vi "main_003_beta.vi"() -> ()   [LabVIEW 2017]
uses:
  ISEGNHQxxu/iseg NHQ VISA Control.ctl
  <vilib>/Analysis/1siggen.llb/Ramp Pattern by Samples.vi
  <vilib>/Utility/file.llb/Read From Spreadsheet File (DBL).vi
  <vilib>/Utility/file.llb/Write Delimited Spreadsheet (string).vi
  <vilib>/Utility/file.llb/Write Delimited Spreadsheet (DBL).vi
  <vilib>/Platform/browser.llb/Open URL in Default Browser (path).vi
  <vilib>/Analysis/NI_AALBase.lvlib
  Newport ESP301/Newport ESP301.lvlib
panel:
  in  "continous acq.":bool
  in  "snap":bool
  in  "dark":bool
  in  "savebin":bool
  in  "savepng":bool
  in  "count?":bool
  in  "dark?":bool
  in  "threshold":i32=100
  in  "t_exp":dbl=0.10000637173652649 caption="Exposure time [s]"
  in  "dark_load":bool
  in  "frames":i32=300
  in  "avg[t] acc[f]":bool
  in  "Value in":dbl=2.0 caption="binning"
  in  "stop":bool
  out "Slide":dbl(slide)=0.9966666666666667 scale=0.0..1.0
  in  "open base path":bool
  in  "Path":path=path "Z:/Ediff/data/2018/08/180807"
  in  "Tab Control":T1(tab)=enum."delayscan"
  out "Waveform Chart":dbl(graph)=8402498.700000005
  in  "array size":i32=50
  out "noise-o-meter":dbl=7.252741087138157 format="%.1g"
  out "Actual Voltage":dbl[unit]=-90.03 format="%.2f"
  in  "volt_set":bool
  in  "Nominal Voltage":sgl=90.0 min=0 max=1000 step=1 format="%.2f"
  out "delayscan_time/step":dbl format="%.2f"
  out "delayscan_steps":i32
  in  "esp_rel_delta_fs":dbl=0.015 caption="delta [fs]" min=0.0
  in  "delayscan_go":bool
  in  "waypoints":string[][](table)=[["-500", "50"], ["500", ""], ["", ""]]
  in  "delayscan_header":string="DelayScan01" caption="header"
  in  "iterations":i32=1
  out "XY Graph":cluster{"Array":dbl[], dbl[]}(graph)={"Array"=[-500.0, -450.0, -400.0, -350.0, -300.0, -250.0, -200.0, -150.0, -100.0, -50.0, 0.0, 50.0, 100.0, 150.0, 200.0, 250.0, 300.0, 350.0, 400.0, 450.0, 500.0], [74.7680418855, 74.77553669695, 0.0, 0.0, 0.0, 0.0, 0.0, 0.0, 0.0, 0.0, 0.0, 0.0, 0.0, 0.0, 0.0, 0.0, 0.0, 0.0, 0.0, 0.0, 0.0]}
  in  "delayscan_stop":bool
  in  "esp_abs_dest":dbl=74.87296924580001 caption="[mm]"
  out "t0 @":dbl=74.84299 format="%.6g"
  in  "esp_set_t0":bool
  in  "esp_abs_time":dbl=200.0 caption="[fs]"
  in  "esp_rel_delta":dbl=0.015 caption="delta [mm]" min=0.0
  in  "esp_abs_go":bool
  in  "esp_rel-":bool
  in  "esp_rel+":bool
  out "delay_pos":dbl=74.77555 caption="[mm]" format="%.6g"
  out "esp_pos_fs":dbl=-449.91125160329966 caption="[fs]" format="%.6g"
  in  "delayscan_pause":bool caption="pause"
  out "duration":dbl format="%<%H:%M:%S>t"
  out "Slide 2":dbl(slide)=0.999 scale=0.0..1.0
  in  "meas_stop_volt":bool
  in  "meas_start_volt":bool
  in  "head":string="PowerVoltScan1"
  in  "volt_start":dbl format="%0.2f"
  in  "volt_end":dbl=1.0 format="%0.2f"
  in  "volt_samples":i32=128
  in  "move2com":bool
  in  "meas_start_XY":bool
  in  "showcom":bool
  in  "VISA ISEG":refnum<visa-resource-name>="COM3"
  in  "Channel (A)":enum16{"A", "B"}(ring)=enum."B"
  out "error out":errorcluster
  in  "volt_timeout":u32=6000
  in  "volt_threshold":sgl=2.0 max=4000 format="%.2f"
  in  "esp_axis":i32=1 caption="ESP Axis" min=1 max=3
  in  "esp_visa":refnum<visa-resource-name>="COM2" caption="ESP VISA"
  out "esp301":errorcluster
  in  "Serial Link (RS232)":enum16{"RS232", "USB"}(ring)
  out "captured":dbl[][](graph)
  out "live":dbl[][](graph)
  in  "close":bool
  # "camera"
  # "voltage supply"
  # "Move absolute"
  # "Move relative"
  # "Axis1"
  # "Axis2"
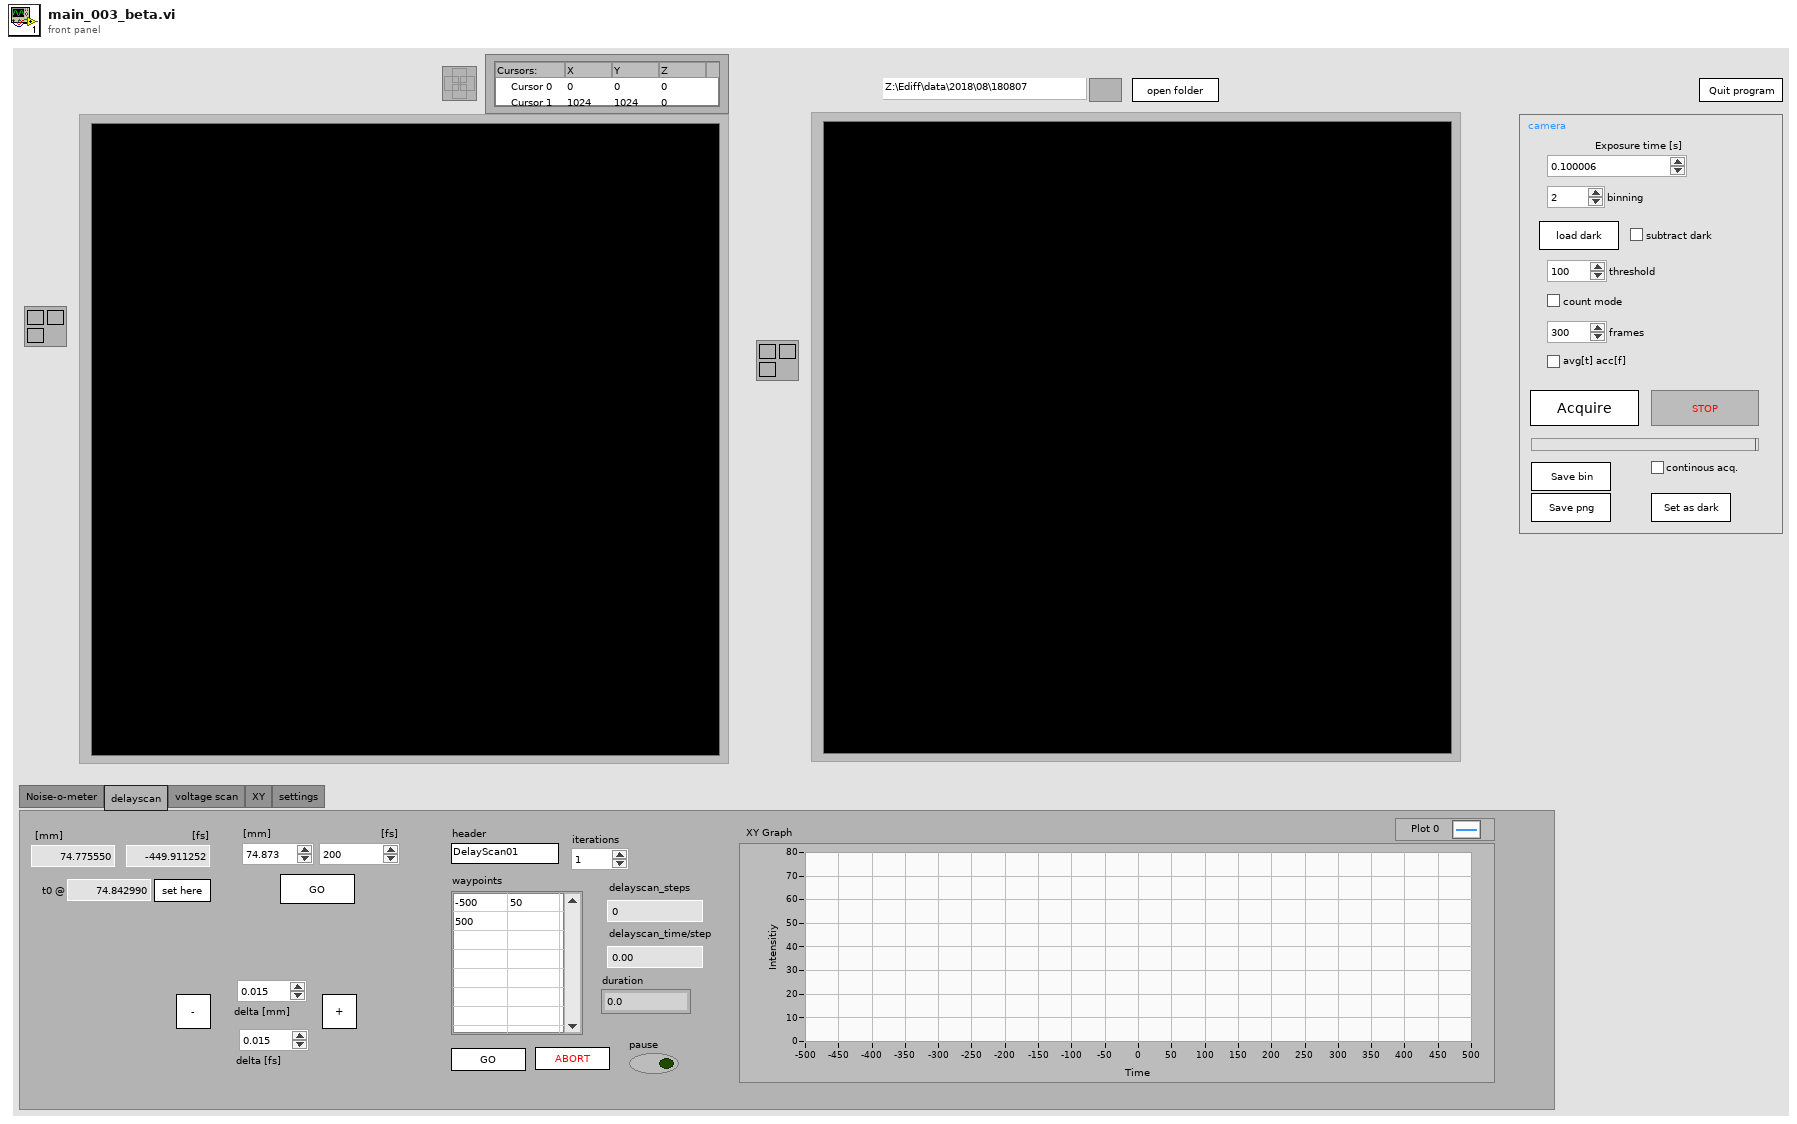
[diagram p1: front panel]
types:
  T1 = enum32{"Noise-o-meter", "delayscan", "voltage scan", "XY", "settings"}
  T2 = typedef "Image Type" = u32
  T3 = typedef "IMAQ Image.ctl" = refnum<image>
  T4 = cluster{"height":u32, "width":u32, "datatype":u32}
  T5 = cluster{"Axis1 moving":bool, "Axis2 moving":bool, "Axis3 moving":bool, "Axis4 moving":bool, "Motor Power of at least one axis":bool, "Reserved":bool, "Reserved":bool, "Reserved":bool, "Axis5 moving 2":bool, "Axis6 moving 2":bool, "Reserved":bool, "Reserved":bool, "Motor Power of at least one axis":bool, "Reserved":bool, "Reserved":bool, "Reserved":bool}
  T6 = typedef "iseg NHQ VISA Control.ctl" = cluster{"VISA Resource Name":refnum<visa-resource-name>, "FP Notation":bool, "Maximum Voltage":u32, "Maximum Current":u32}
  T7 = typedef "LVCursorListTypeDef.ctl" = cluster{"Name":string, "Color":u32, "Style":u8, "Point Style":u8, "Name Visible":bool, "Allow Drag":bool, "Cursor Mode":u32, "Plot":i32, "Index":i32, "Position":cluster{"X":dbl, "Y":dbl}, "X Scale":u32, "Y Scale":u32, "Watch Plots":i32[], "Watch All Plots":bool, "Plot Area":i32, "Label Offset":cluster{"X":dbl, "Y":dbl}}[]
  T8 = cluster{"Name":string, "Color":u32, "Style":u8, "Point Style":u8, "Name Visible":bool, "Allow Drag":bool, "Cursor Mode":u32, "Plot":i32, "Index":i32, "Position":cluster{"X":dbl, "Y":dbl}, "X Scale":u32, "Y Scale":u32, "Watch Plots":i32[], "Watch All Plots":bool, "Plot Area":i32, "Label Offset":cluster{"X":dbl, "Y":dbl}}
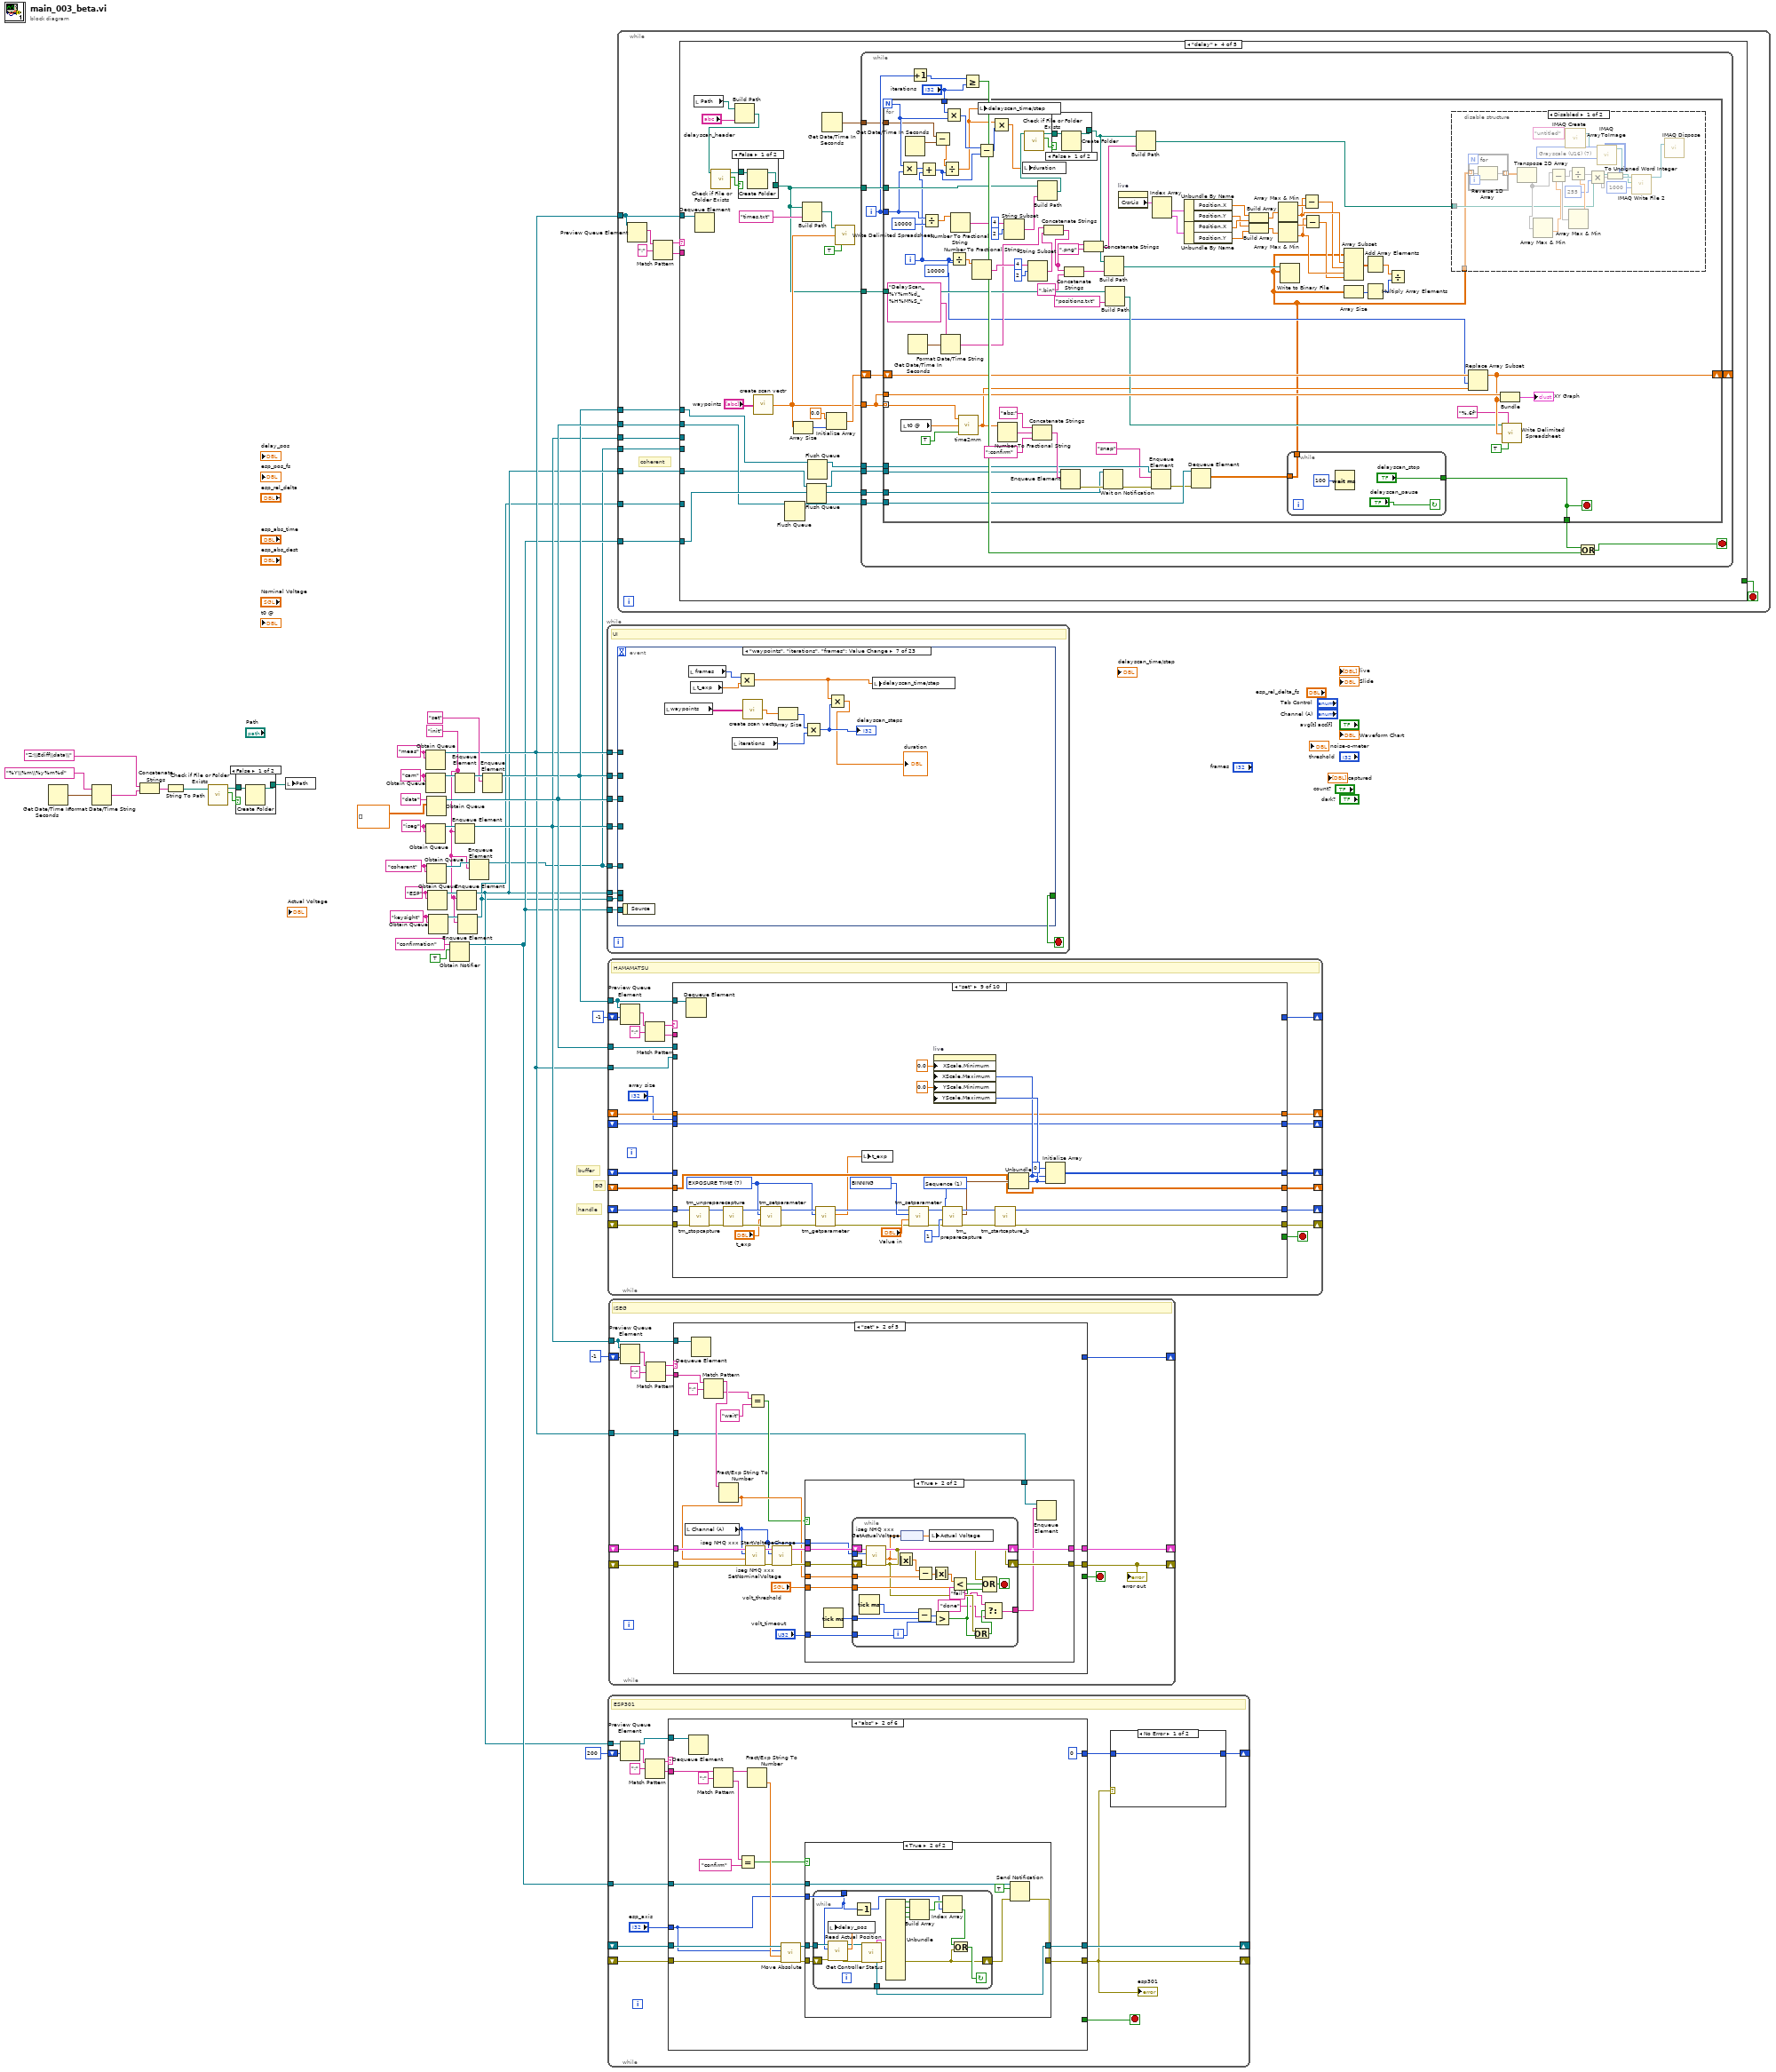
[diagram p0: block diagram]
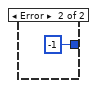
[diagram p3: hidden frame]
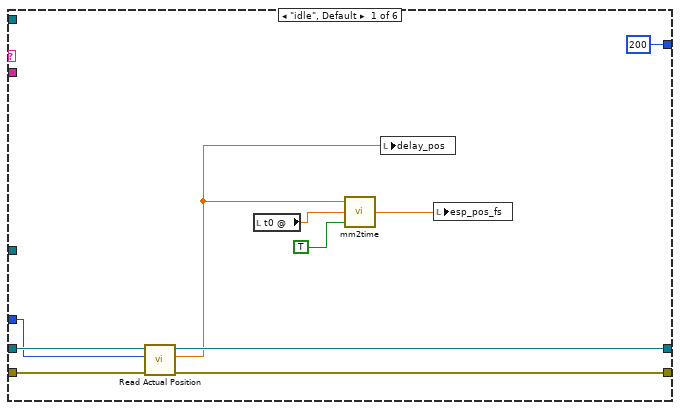
[diagram p4: hidden frame]
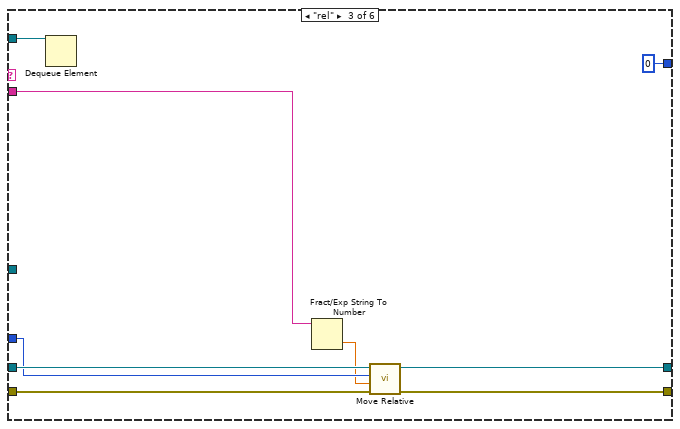
[diagram p6: hidden frame]
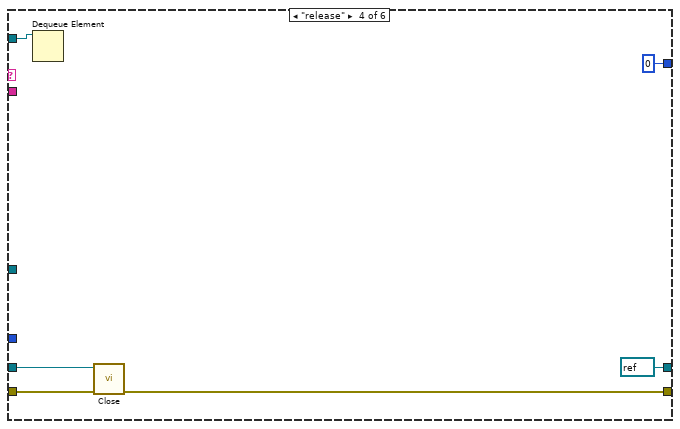
[diagram p7: hidden frame]
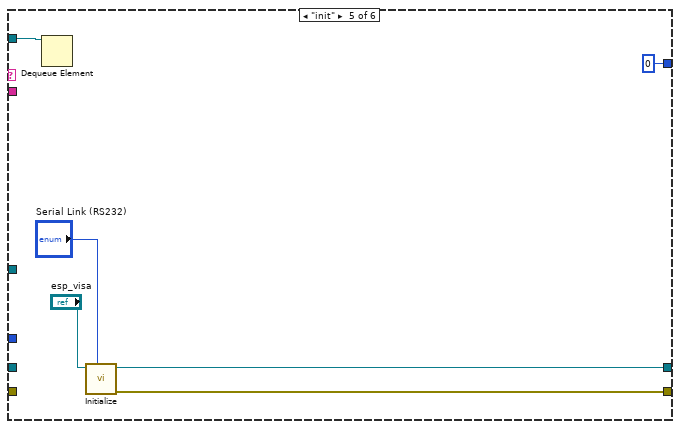
[diagram p8: hidden frame]
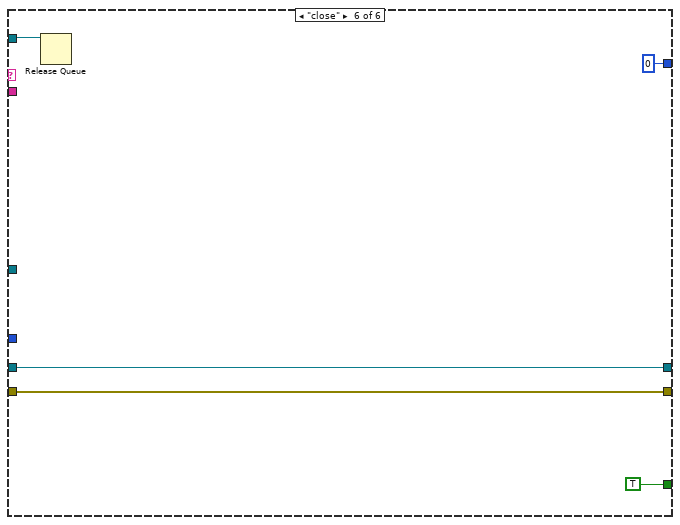
[diagram p9: hidden frame]
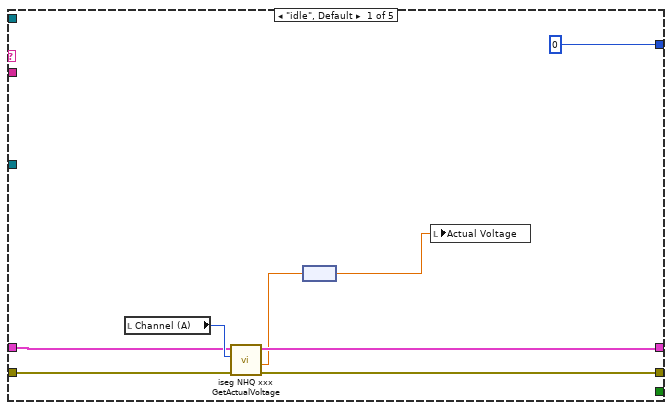
[diagram p10: hidden frame]
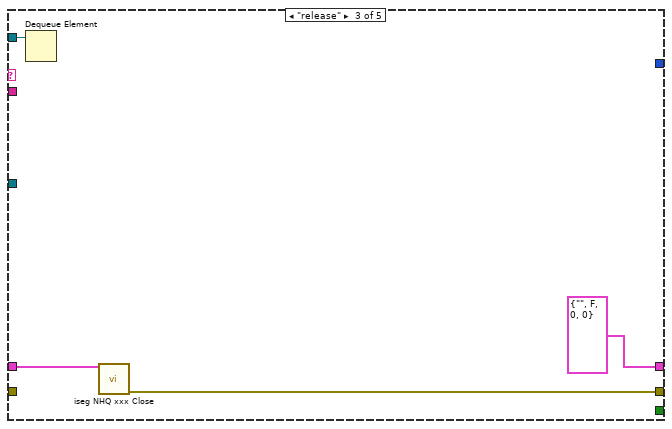
[diagram p12: hidden frame]
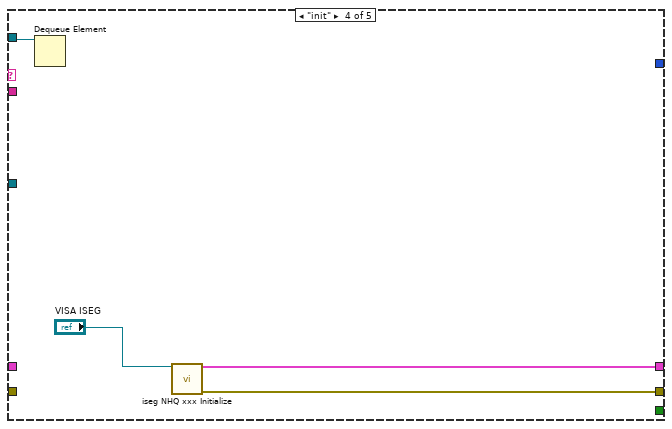
[diagram p13: hidden frame]
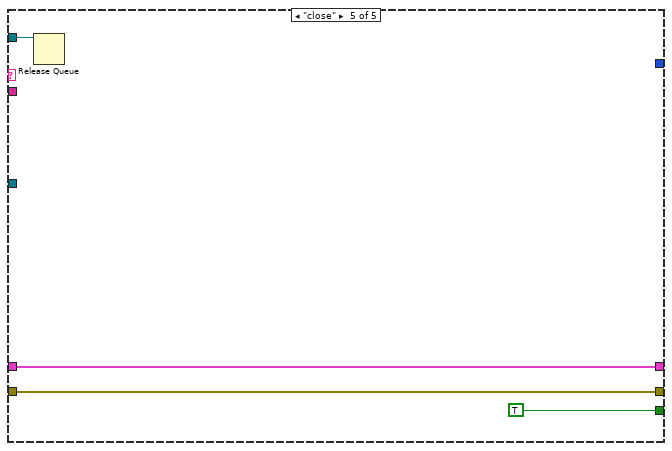
[diagram p14: hidden frame]
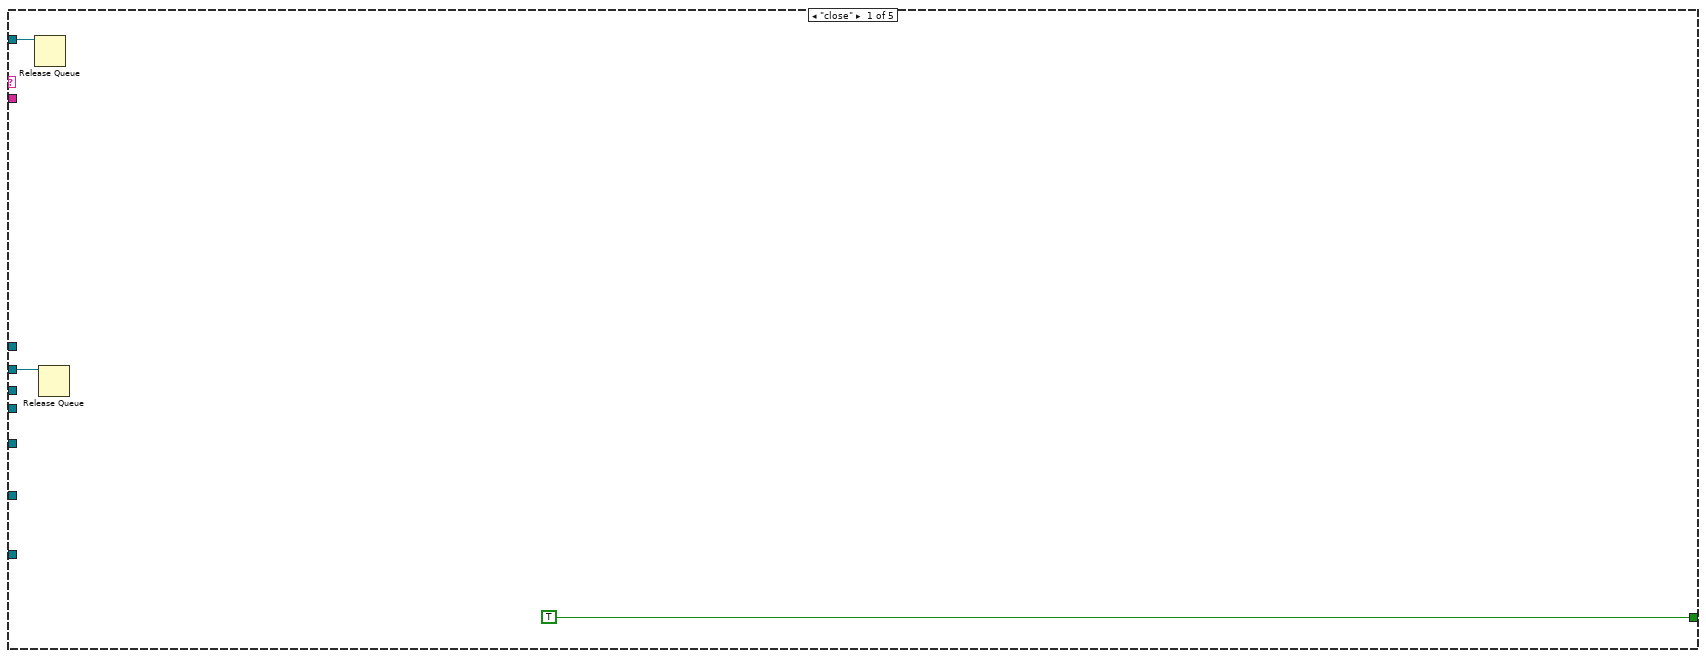
[diagram p15: hidden frame]
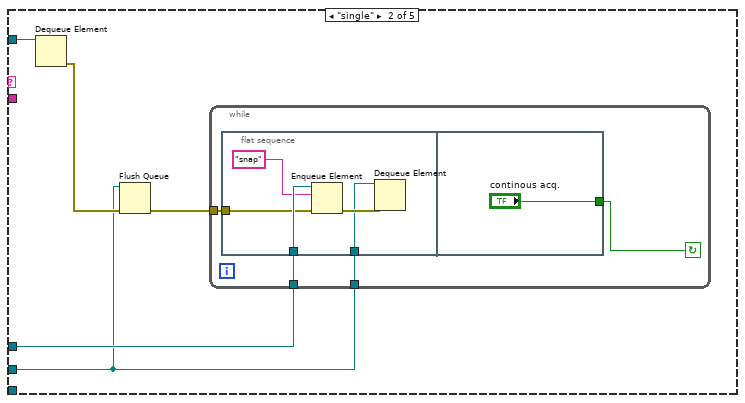
[diagram p16: hidden frame]
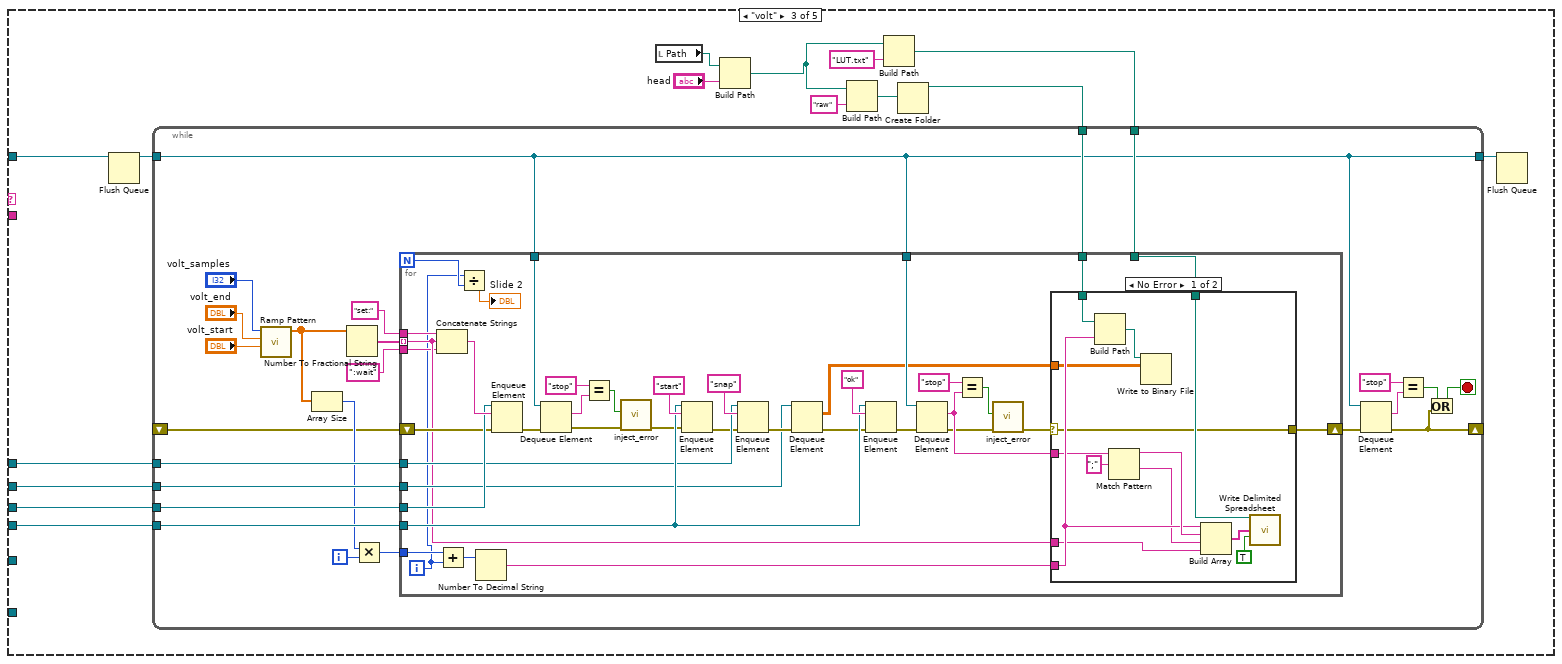
[diagram p17: hidden frame]
diagram:
  w3 = "keysight" ("name (unnamed)")
  w19 = "ESP" ("name (unnamed)")
  w24 = "coherent" ("name (unnamed)")
  w28 = "iseg" ("name (unnamed)")
  w2 = "init" ("element")
  w35 = "meas" ("name (unnamed)")
  w36 = "cam" ("name (unnamed)")
  # "BG"
  # "handle"
  # "buffer"
  n1 = Get Date/Time In Seconds() -> (seconds since 1Jan1904=w16:timestamp)
  n2 = Format Date/Time String(time format string (%c)="%Y\\%m\\%y%m%d", seconds (now)=w16) -> (date/time string=w14:string)  [unwired: 1 in]
  n3 = Concatenate Strings("Z:\\Ediff\\data\\" ("string"), w14) -> (w12:string)
  n4 = String To Path(string=w12) -> (path=w9:path)
  n5 = call <vilib>:"Check if File or Folder Exists.vi"("path"=w9) -> ("file or folder exists?"=w11:bool, "dup path"=w10:path)  [unwired: 8 in, 1 out]
  n6 = case shown="False" w11 {
    tunnel: [w40 w41] -> w8
    tunnel: w10 -> [w39 w41]
    frame False {
      n7 = Create Folder(path (use dialog)=w39) -> (created path=w40:path)  [unwired: 2 in, 2 out]
    }
    frame True {
    }
  }
  n8 = local write "Path"(w8) -> ()
  n9 = Obtain Queue(name (unnamed)=w35, element data type=w35) -> (queue out=w23:refnum<queue>)  [unwired: 3 in, 2 out]
  n10 = Obtain Queue(name (unnamed)=w36, element data type=w36) -> (queue out=w38:refnum<queue>)  [unwired: 3 in, 2 out]
  n11 = Obtain Queue(name (unnamed)=w28, element data type=w28) -> (queue out=w27:refnum<queue>)  [unwired: 3 in, 2 out]
  n12 = Obtain Queue(name (unnamed)="data", element data type=dbl[][] []) -> (queue out=w31:refnum<queue>)  [unwired: 3 in, 2 out]
  n13 = Obtain Queue(name (unnamed)=w24, element data type=w24) -> (queue out=w7:refnum<queue>)  [unwired: 3 in, 2 out]
  n14 = Obtain Queue(name (unnamed)=w19, element data type=w19) -> (queue out=w18:refnum<queue>)  [unwired: 3 in, 2 out]
  n15 = Obtain Queue(name (unnamed)=w3, element data type=w3) -> (queue out=w4:refnum<queue>)  [unwired: 3 in, 2 out]
  n16 = Obtain Notifier(name (unnamed)="confirmation", notification data type=TRUE) -> (notifier out=w20:refnum<notifier>)  [unwired: 2 in, 2 out]
  n17 = Enqueue Element(queue=w38, element=w2) -> (queue out=w34:refnum<queue>)  [unwired: 2 in, 2 out]
  n18 = Enqueue Element(queue=w27, element=w2) -> (queue out=w25:refnum<queue>)  [unwired: 2 in, 2 out]
  n19 = Enqueue Element(queue=w18, element=w2) -> (queue out=w17:refnum<queue>)  [unwired: 2 in, 2 out]
  n20 = Enqueue Element(queue=w4, element=w2) -> (queue out=w1:refnum<queue>)  [unwired: 2 in, 2 out]
  n21 = Enqueue Element(queue=w7, element=w2) -> (queue out=w6:refnum<queue>)  [unwired: 2 in, 2 out]
  n22 = Enqueue Element(queue=w34, element="set") -> (queue out=w30:refnum<queue>)  [unwired: 2 in, 2 out]
  n23 = while {
    tunnel: w30 -> [w50]
    tunnel: w23 -> [w49]
    tunnel: w31 -> [w48]
    tunnel: w25 -> [w46]
    tunnel: w6 -> [w45]
    tunnel: w20 -> [w44]
    tunnel: w17 -> [w43]
    tunnel: w1 -> [w42]
    stop <- w47 stop-if-true
    # "UI"
    n24 = event shown="[6] \"waypoints\", \"iterations\", \"frames\": Value Change" {
      selector: _ -> [_ _ _ _ _ _ _ _ _ _ _ _ _ _ _ _ _ _ _ _ _ _ _]
      dyn-events: _ -> [_ _ _ _ _ _ _ _ _ _ _ _ _ _ _ _ _ _ _ _ _ _ _]
      timeout: _ -> [_ _ _ _ _ _ _ _ _ _ _ _ _ _ _ _ _ _ _ _ _ _ _]
      tunnel: w50 -> [_ w65 _ _ _ _ _ _ _ _ _ w108 w110 _ _ _ _ _ _ w161 _ _ _]
      tunnel: w49 -> [_ w66 _ _ _ _ _ _ _ w102 _ _ _ w111 w114 w115 _ _ w155 _ w168 w170 _]
      tunnel: w48 -> [_ _ _ _ _ _ _ _ _ _ _ _ _ _ _ _ _ _ _ _ _ _ _]
      tunnel: [_ TRUE _ _ _ _ _ _ _ _ _ _ _ _ _ _ _ _ _ _ _ _ _] -> w47
      tunnel: w46 -> [_ w62 _ _ _ _ _ _ _ _ _ _ _ _ _ _ _ _ _ _ _ _ w175]
      tunnel: w45 -> [_ w59 _ _ _ _ _ _ _ _ _ _ _ _ _ _ _ _ _ _ _ _ _]
      tunnel: w44 -> [_ w56 _ _ _ _ _ _ _ _ _ _ _ _ _ _ _ _ _ _ _ _ _]
      tunnel: w43 -> [_ w58 w72 w77 _ _ _ _ _ _ _ _ _ _ _ _ _ _ _ _ _ _ _]
      tunnel: w42 -> [_ w51 _ _ _ _ _ _ _ _ _ _ _ _ _ _ _ _ _ _ _ _ _]
      event Timeout {
        n25 = event-data() -> ()  [unwired: 1 in, 1 out]
      }
      event "close": Value Change {
        w54 = "close" ("element")
        w55 = "release" ("element")
        n26 = event-data() -> ()  [unwired: 1 in, 1 out]
        n27 = Enqueue Element(queue=w59, element=w55) -> (queue out=w60:refnum<queue>)  [unwired: 2 in, 2 out]
        n28 = Enqueue Element(queue=w58, element=w55) -> (queue out=w57:refnum<queue>)  [unwired: 2 in, 2 out]
        n29 = Enqueue Element(queue=w62, element=w55) -> (queue out=w61:refnum<queue>)  [unwired: 2 in, 2 out]
        n30 = Enqueue Element(queue=w65, element=w55) -> (queue out=w64:refnum<queue>)  [unwired: 2 in, 2 out]
        n31 = Enqueue Element(queue=w66, element=w54) -> ()  [unwired: 2 in, 3 out]
        n32 = Enqueue Element(queue=w64, element=w54) -> ()  [unwired: 2 in, 3 out]
        n33 = Enqueue Element(queue=w61, element=w54) -> ()  [unwired: 2 in, 3 out]
        n34 = Enqueue Element(queue=w60, element=w54) -> ()  [unwired: 2 in, 3 out]
        n35 = Enqueue Element(queue=w57, element=w54) -> ()  [unwired: 2 in, 3 out]
        n36 = Release Notifier(notifier=w56) -> ()  [unwired: 2 in, 3 out]
        n37 = Flush Queue(queue=w51) -> (queue out=w52:refnum<queue>)  [unwired: 1 in, 2 out]
        n38 = Enqueue Element(queue=w52, element=w55) -> (queue out=w53:refnum<queue>)  [unwired: 2 in, 2 out]
        n39 = Enqueue Element(queue=w53, element=w54) -> ()  [unwired: 2 in, 3 out]
      }
      event "esp_abs_go": Value Change {
        n40 = event-data() -> ()  [unwired: 1 in, 1 out]
        n41 = local read "esp_abs_dest"() -> (w68:dbl)
        n42 = Number To Fractional String(number=w68) -> (F-format string=w69:string)  [unwired: 3 in]
        n43 = Concatenate Strings("abs:" ("string"), w69, ":confirm" ("string")) -> (w71:string)
        n44 = Enqueue Element(queue=w72, element=w71) -> ()  [unwired: 2 in, 3 out]
      }
      event "esp_rel+", "esp_rel-": Value Change {
        n45 = event-data() -> ()  [unwired: 1 in, 1 out]
        n46 = local read "esp_rel_delta"() -> (w75:dbl)
        n47 = Negate(x=w75) -> (-x=w76:dbl)
        n48 = Select(t=w76, s="esp_rel-", f=w75) -> (s? t:f=w74:dbl)
        n49 = Number To Fractional String(number=w74) -> (F-format string=w79:string)  [unwired: 3 in]
        n50 = Concatenate Strings("rel:" ("string"), w79) -> (w78:string)
        n51 = Enqueue Element(queue=w77, element=w78) -> ()  [unwired: 2 in, 3 out]
      }
      event "esp_rel_delta_fs": Value Change {
        n52 = event-data() -> ()  [unwired: 1 in, 1 out]
        n53 = local read "esp_rel_delta_fs"() -> (w81:dbl)
        n54 = call "time2mm.vi"("fs[1]/ps[0]"=TRUE, "time"=w81) -> ("position (mm)"=w82:dbl)  [unwired: 1 in]
        n55 = local write "esp_rel_delta"(w82) -> ()
      }
      event "esp_rel_delta": Value Change {
        n56 = event-data() -> ()  [unwired: 1 in, 1 out]
        n57 = local read "esp_rel_delta"() -> (w85:dbl)
        n58 = call "mm2time.vi"("fs?"=TRUE, "distance (mm)"=w85) -> ("time in fs/ps seconds"=w84:dbl)  [unwired: 1 in]
        n59 = local write "esp_rel_delta_fs"(w84) -> ()
      }
      event "waypoints", "iterations", "frames": Value Change {
        n60 = event-data() -> ()  [unwired: 1 in, 1 out]
        n61 = local read "waypoints"() -> (w95:string[][])
        n62 = local read "frames"() -> (w90:i32)
        n63 = local read "t_exp"() -> (w89:dbl)
        n64 = local read "iterations"() -> (w92:i32)
        n65 = Multiply(x=w90, y=w89) -> (x*y=w88:dbl)
        n66 = call "create scan vectr.vi"("Table Control"=w95) -> ("Array"=w94:dbl[])
        n67 = Array Size(array=w94) -> (size(s)=w93:i32)
        n68 = Multiply(x=w93, y=w92) -> (x*y=w91:i32)
        "delayscan_steps" <- w91
        n69 = Multiply(x=w88, y=w91) -> (x*y=→"duration":dbl)
        n70 = local write "delayscan_time/step"(w88) -> ()
      }
      event "esp_set_t0": Value Change {
        n71 = event-data() -> ()  [unwired: 1 in, 1 out]
        n72 = local read "delay_pos"() -> (w96:dbl)
        n73 = local write "t0 @"(w96) -> ()
      }
      event "esp_abs_time": Value Change {
        n74 = event-data() -> ()  [unwired: 1 in, 1 out]
        n75 = local read "esp_abs_time"() -> (w97:dbl)
        n76 = local read "t0 @"() -> (w98:dbl)
        n77 = call "time2mm.vi"("fs[1]/ps[0]"=TRUE, "Offset (mm)"=w98, "time"=w97) -> ("position (mm)"=w99:dbl)
        n78 = local write "esp_abs_dest"(w99) -> ()
      }
      event "delayscan_go": Value Change {
        n79 = event-data() -> ()  [unwired: 1 in, 1 out]
        n80 = Enqueue Element(queue=w102, element="delay") -> ()  [unwired: 2 in, 3 out]
      }
      event "esp_abs_dest": Value Change {
        n81 = event-data() -> ()  [unwired: 1 in, 1 out]
        n82 = local read "esp_abs_dest"() -> (w106:dbl)
        n83 = local read "t0 @"() -> (w105:dbl)
        n84 = call "mm2time.vi"("fs?"=TRUE, "Offset (mm)"=w105, "distance (mm)"=w106) -> ("time in fs/ps seconds"=w103:dbl)
        n85 = local write "esp_abs_time"(w103) -> ()
      }
      event "dark": Value Change {
        n86 = event-data() -> ()  [unwired: 1 in, 1 out]
        n87 = Enqueue Element(queue=w108, element="dark") -> ()  [unwired: 2 in, 3 out]
      }
      event "t_exp": Value Change {
        n88 = event-data() -> ()  [unwired: 1 in, 1 out]
        n89 = Enqueue Element(queue=w110, element="set") -> ()  [unwired: 2 in, 3 out]
      }
      event "snap": Value Change {
        n90 = event-data() -> ()  [unwired: 1 in, 1 out]
        n91 = Enqueue Element(queue=w111, element="single") -> ()  [unwired: 2 in, 3 out]
      }
      event "meas_start_volt": Value Change {
        n92 = event-data() -> ()  [unwired: 1 in, 1 out]
        n93 = Enqueue Element(queue=w114, element="volt") -> ()  [unwired: 2 in, 3 out]
      }
      event "meas_stop_volt": Value Change {
        n94 = event-data() -> ()  [unwired: 1 in, 1 out]
        n95 = Enqueue Element(queue=w115, element="stop") -> ()  [unwired: 2 in, 3 out]
      }
      event "open base path": Value Change {
        n96 = event-data() -> ()  [unwired: 1 in, 1 out]
        n97 = local read "Path"() -> (w117:path)
        n98 = call-poly <vilib>:"Open URL in Default Browser.vi"("path"=w117) -> ()  [unwired: 5 in, 2 out]
      }
      event "savebin", "savepng": Value Change {
        n99 = event-data() -> ()  [unwired: 1 in, 1 out]
        n100 = Get Date/Time In Seconds() -> (seconds since 1Jan1904=w123:timestamp)
        n101 = local read "Path"() -> (w119:path)
        n102 = Format Date/Time String(time format string (%c)="MCPIMG_%Y%m%d_%H%M%S", seconds (now)=w123) -> (date/time string=w118:string)  [unwired: 1 in]
        n103 = local read "captured"() -> (w120:dbl[][])
        n104 = case shown="False" "savebin" {
          tunnel: w120 -> [w138 w154]
          tunnel: w119 -> [w135 w148]
          tunnel: w118 -> [w133 w149]
          frame False {
            w143 = T2 7 items=["Grayscale (U8)", "Grayscale (I16)", "Grayscale (SGL)", "Complex (CSG)", "RGB (U32)", "HSL (U32)", "RGB (U64)", "Grayscale (U16)"] ("Image Type")
            n105 = for {
              tunnel: w138 -> [w146] mode=indexing
              tunnel: [w145] -> w137 mode=indexing
              n106 = Reverse 1D Array(array=w146) -> (reversed array=w145:dbl[])
            }
            n107 = Concatenate Strings(w133, ".png" ("string")) -> (w134:string)
            n108 = Transpose 2D Array(2D array=w137) -> (transposed array=w126:dbl[][])
            n109 = Array Max & Min(array=w126) -> (min value=w125:dbl)  [unwired: 3 out]
            n110 = Build Path(base path=w135, name or relative path=w134) -> (appended path=w136:path)
            n111 = Subtract(x=w126, y=w125) -> (x-y=w124:dbl[][])
            n112 = call "IMAQ Create"("Image Name"="untitled", "Image Type"=w143) -> ("New Image"=w144:T3)  [unwired: 3 in, 1 out]
            n113 = Array Max & Min(array=w124) -> (max value=w131:dbl)  [unwired: 3 out]
            n114 = Divide(x=w124, y=w131) -> (x/y=w130:dbl[][])
            n115 = Multiply(x=w130, y=255) -> (x*y=w128:dbl[][])
            n116 = To Unsigned Word Integer(number=w128) -> (unsigned 16bit integer=w127:u16[][])
            n117 = call "IMAQ ArrayToImage"("Image Pixels (U16)"=w127, "Image"=w144) -> ("Image Out"=w142:T3)  [unwired: 8 in, 1 out]
            n118 = call-poly "IMAQ Write File 2"("Image Quality"=u32 1000, "File Path"=w136, "Image"=w142) -> ("Image Out (duplicate)"=w140:T3)  [unwired: 7 in, 1 out]
            n119 = call "IMAQ Dispose"("Image"=w140) -> ()  [unwired: 5 in, 1 out]
          }
          frame True {
            n120 = Concatenate Strings(w149, ".bin" ("string")) -> (w151:string)
            n121 = Build Path(base path=w148, name or relative path=w151) -> (appended path=w147:path)
            n122 = Write to Binary File(file (use dialog)=w147, data=w154) -> (refnum out=w153:refnum<file>, error out=w152:errorcluster)  [unwired: 4 in, 1 out]
            n123 = Close File(refnum=w153, error in=w152) -> ()  [unwired: 2 out]
          }
        }
      }
      event "meas_start_XY": Value Change {
        n124 = event-data() -> ()  [unwired: 1 in, 1 out]
        n125 = Enqueue Element(queue=w155, element="XY") -> ()  [unwired: 2 in, 3 out]
      }
      event "dark_load": Value Change {
        n126 = event-data() -> ()  [unwired: 1 in, 1 out]
        n127 = local read "Path"() -> (w160:path)
        n128 = call "File Dialog"("start path"=w160) -> ("selected path"=w158:path, "cancelled"=w157:bool)  [unwired: 11 in, 2 out]
        n129 = case shown="False" w157 {
          tunnel: w161 -> [w166 _]
          tunnel: "dark_load:" ("element") -> [w164 _]
          tunnel: w158 -> [w162 _]
          frame False {
            n130 = Path To String(path=w162) -> (string=w163:string)
            n131 = Concatenate Strings(w164, w163) -> (w165:string)
            n132 = Enqueue Element(queue=w166, element=w165) -> ()  [unwired: 2 in, 3 out]
          }
          frame True {
          }
        }
      }
      event "move2com": Value Change {
        n133 = event-data() -> ()  [unwired: 1 in, 1 out]
        n134 = Enqueue Element(queue=w168, element="mov2cursor") -> ()  [unwired: 2 in, 3 out]
      }
      event "showcom": Value Change {
        n135 = event-data() -> ()  [unwired: 1 in, 1 out]
        n136 = Enqueue Element(queue=w170, element="showcom") -> ()  [unwired: 2 in, 3 out]
      }
      event "volt_set": Value Change {
        n137 = event-data() -> ()  [unwired: 1 in, 6 out]
        n138 = local read "Nominal Voltage"() -> (w171:sgl)
        n139 = Number To Fractional String(number=w171) -> (F-format string=w172:string)  [unwired: 3 in]
        n140 = Concatenate Strings("set:" ("element"), w172) -> (w174:string)
        n141 = Enqueue Element(queue=w175, element=w174) -> ()  [unwired: 2 in, 3 out]
      }
    }
  }
  n142 = while {
    tunnel: w30 -> [w194]
    shift-right: [w192] -> _
    shift-left: _ -> [w191]
    shift-right: [w190] -> _
    shift-left: _ -> [w189]
    shift-right: [w188] -> _
    shift-left: _ -> [w187]
    shift-right: [w186] -> _
    shift-left: _ -> [w185]
    shift-right: [w183] -> _
    shift-left: -1 -> [w184]
    tunnel: w31 -> [w182]
    tunnel: w23 -> [w181]
    shift-right: [w180] -> _
    shift-left: _ -> [w179]
    shift-right: [w177] -> _
    shift-left: _ -> [w178]
    stop <- w193 stop-if-true
    # "HAMAMATSU"
    n143 = Preview Queue Element(queue=w194, timeout in ms (-1)=w184) -> (element=w198:string)  [unwired: 1 in, 3 out]
    n144 = Match Pattern(string=w198, regular expression=":") -> (before substring=w196:string, after substring=w195:string)  [unwired: 1 in, 2 out]
    n145 = case shown="\"set\"" w196 {
      tunnel: w195 -> [_ _ w298 _ _ w388 _ _ _ _]
      tunnel: w194 -> [_ w237 w299 w333 w382 w392 w404 w407 w433 w455]
      tunnel: [_ _ _ _ _ _ _ _ _ TRUE] -> w193
      tunnel: [w217 w239 w302 w338 w380 w389 w396 w412 w421 w450] -> w192
      tunnel: w191 -> [w219 w242 w304 w340 w380 w389 w400 _ w447 w450]
      tunnel: [w218 w234 w303 w337 w379 w390 u32 0 ("Handle out") w410 w422 w451] -> w190
      tunnel: w189 -> [w220 w240 w305 w341 w379 w390 w401 _ w445 w451]
      tunnel: [w216 w241 w297 w336 w381 w391 w402 w408 w434 w452] -> w188
      tunnel: w187 -> [w216 w241 w297 w336 w381 w391 w402 w408 _ w452]
      tunnel: [w215 w238 w306 w339 w378 w385 w403 w409 w425 w453] -> w186
      tunnel: w185 -> [w215 w238 w306 w339 _ _ w403 w409 w425 w453]
      tunnel: [0 _ _ _ _ _ _ _ _ _] -> w183
      tunnel: w182 -> [_ w233 w307 _ _ _ _ _ _ _]
      tunnel: w181 -> [_ _ _ w334 _ _ _ _ _ _]
      tunnel: [w201 w228 w301 w325 w377 w384 w394 w406 w427 w449] -> w180
      tunnel: w179 -> [w210 w231 w301 w328 w377 w384 w394 w406 w427 w449]
      tunnel: w178 -> [w205 w230 w300 w326 w376 w383 w393 w405 w426 w448]
      tunnel: [w204 w227 w300 w324 w376 w383 w393 w405 w426 w448] -> w177
      tunnel: "array size" -> [w203 w229 _ w327 _ _ _ _ _ _]
      frame "idle", Default {
        n146 = local read "threshold"() -> (w221:i32)
        n147 = call "tm_getnextframe_a.vi"("error in (no error)"=w219, "Buffer"=w216, "Handle in"=w220) -> ("error out"=w217:errorcluster, "Data"=w211:u16[][], "Handle out"=w218:u32)  [unwired: 6 in]
        n148 = local read "dark?"() -> (w222:bool)
        n149 = local read "count?"() -> (w212:bool)
        n150 = case shown="False" w222 {
          tunnel: [w223 w226] -> w213
          tunnel: w211 -> [w223 w225]
          tunnel: w215 -> [_ w224]
          frame False {
          }
          frame True {
            n151 = Subtract(x=w225, y=w224) -> (x-y=w226:dbl[][])
          }
        }
        n152 = call "filtr_b.vi"("count?"=w212, "threshold"=w221, "input array"=w213) -> ("output array"=w199:dbl[][])  [unwired: 8 in]
        n153 = Add Array Elements(numeric array=w199) -> (sum=w200:dbl)
        n154 = call "ringbuffer.vi"("new val"=w200, "index in"=w205, "array size"=w203, "array in"=w210) -> ("index out"=w204:i32, "array out"=w201:dbl[])  [unwired: 6 in]
        n155 = local write "live"(w199) -> ()
        n156 = local write "Waveform Chart"(w200) -> ()
        n157 = call <vilib>:"Std Deviation and Variance.vi"("X"=w201) -> ("mean"=w206:dbl, "standard deviation"=w209:dbl)  [unwired: 1 in, 1 out]
        n158 = Divide(x=w209, y=w206) -> (x/y=w208:dbl)
        n159 = Multiply(x=w208, y=100.0) -> (x*y=w202:dbl)
        n160 = local write "noise-o-meter"(w202) -> ()
      }
      frame "snap" {
        n161 = Dequeue Element(queue=w237) -> ()  [unwired: 2 in, 4 out]
        n162 = local read "avg[t] acc[f]"() -> (w236:bool)
        n163 = local read "threshold"() -> (w244:i32)
        n164 = local read "frames"() -> (w243:i32)
        n165 = local read "count?"() -> (w235:bool)
        n166 = local read "dark?"() -> (w245:bool)
        n167 = for {
          N: w243 -> [w263]
          tunnel: w245 -> [w277]
          tunnel: w241 -> [w275]
          tunnel: w240 -> [w276]
          tunnel: w244 -> [w269]
          tunnel: [w273] -> w234
          shift-right: [w272] -> w239
          shift-left: w242 -> [w274]
          tunnel: w238 -> [w268]
          shift-right: [w246] -> w232
          shift-left: w241 -> [w266]
          tunnel: w236 -> [w267]
          tunnel: w235 -> [w265]
          shift-right: [w256] -> w228
          shift-left: w231 -> [w257]
          tunnel: w229 -> [w254]
          shift-right: [w253] -> w227
          shift-left: w230 -> [w255]
          shift-right: [w249] -> _
          shift-left: _ -> [w250]
          i -> [w264]
          stop <- "stop" stop-if-true
          n168 = call "tm_getnextframe_a.vi"("error in (no error)"=w274, "Buffer"=w275, "Handle in"=w276) -> ("error out"=w272:errorcluster, "Data"=w271:u16[][], "Handle out"=w273:u32)  [unwired: 6 in]
          n169 = Divide(x=w264, y=w263) -> (x/y=w262:dbl)
          n170 = case shown="True" w277 {
            tunnel: [w288 w291] -> w270
            tunnel: w271 -> [w288 w290]
            tunnel: w268 -> [_ w289]
            frame False {
            }
            frame True {
              n171 = Subtract(x=w290, y=w289) -> (x-y=w291:dbl[][])
            }
          }
          n172 = local write "Slide"(w262) -> ()
          n173 = Tick Count (ms)() -> (millisecond timer value=w249:u32)
          n174 = call "filtr_b.vi"("count?"=w265, "threshold"=w269, "input array"=w270) -> ("output array"=w248:dbl[][])  [unwired: 8 in]
          n175 = Subtract(x=w249, y=w250) -> ()  [unwired: 1 out]
          n176 = Add Array Elements(numeric array=w248) -> (sum=w247:dbl)
          n177 = call "ringbuffer.vi"("new val"=w247, "index in"=w255, "array size"=w254, "array in"=w257) -> ("index out"=w253:i32, "array out"=w256:dbl[])  [unwired: 6 in]
          n178 = call <vilib>:"Std Deviation and Variance.vi"("X"=w256) -> ("mean"=w258:dbl, "standard deviation"=w260:dbl)  [unwired: 1 in, 1 out]
          n179 = local write "live"(w248) -> ()
          n180 = local write "Waveform Chart"(w247) -> ()
          n181 = Divide(x=w260, y=w258) -> (x/y=w252:dbl)
          n182 = case shown="True" w267 {
            tunnel: w266 -> [w280 w287]
            tunnel: w248 -> [w279 w285]
            tunnel: [w278 w281] -> w246
            tunnel: w264 -> [_ w282]
            frame False {
              n183 = Add(x=w280, y=w279) -> (x+y=w278:dbl[][])
            }
            frame True {
              n184 = Multiply(x=w287, y=w282) -> (x*y=w286:dbl[][])
              n185 = Increment(x=w282) -> (x+1=w283:i32)
              n186 = Add(x=w286, y=w285) -> (x+y=w284:dbl[][])
              n187 = Divide(x=w284, y=w283) -> (x/y=w281:dbl[][])
            }
          }
          n188 = Multiply(x=w252, y=100.0) -> (x*y=w251:dbl)
          n189 = local write "noise-o-meter"(w251) -> ()
          n190 = local write "captured"(w246) -> ()
        }
        n191 = local write "captured"(w232) -> ()
        n192 = Enqueue Element(queue=w233, element=w232) -> ()  [unwired: 2 in, 3 out]
      }
      frame "single" {
        n193 = Dequeue Element(queue=w299) -> ()  [unwired: 2 in, 4 out]
        n194 = Decimal String To Number(string=w298) -> (number=w293:i32)  [unwired: 2 in, 1 out]
        n195 = To Unsigned Quad Integer(1:w297) -> (0:w296:u64[][])
        n196 = for {
          N: w293 -> [_]
          tunnel: w297 -> [w319]
          tunnel: w305 -> [w318]
          tunnel: w304 -> [w317]
          tunnel: [w316] -> w303
          tunnel: [w315] -> w302
          shift-right: [w312] -> w295
          shift-left: w296 -> [w314]
          n197 = call "tm_getnextframe_a.vi"("error in (no error)"=w317, "Buffer"=w319, "Handle in"=w318) -> ("error out"=w315:errorcluster, "Data"=w313:u16[][], "Handle out"=w316:u32)  [unwired: 6 in]
          n198 = Add(x=w313, y=w314) -> (x+y=w312:u64[][])
        }
        n199 = local read "dark?"() -> (w308:bool)
        n200 = Divide(x=w295, y=w293) -> (x/y=w294:dbl[][])
        n201 = case shown="True" w308 {
          tunnel: [w320 w323] -> w311
          tunnel: w294 -> [w320 w322]
          tunnel: w306 -> [_ w321]
          frame False {
          }
          frame True {
            n202 = Subtract(x=w322, y=w321) -> (x-y=w323:dbl[][])
          }
        }
        n203 = local read "threshold"() -> (w309:i32)
        n204 = local read "count?"() -> (w310:bool)
        n205 = call "filtr_b.vi"("count?"=w310, "threshold"=w309, "input array"=w311) -> ("output array"=w292:dbl[][])  [unwired: 8 in]
        n206 = Enqueue Element(queue=w307, element=w292) -> ()  [unwired: 2 in, 3 out]
        n207 = local write "captured"(w292) -> ()
      }
      frame "snap_I" {
        n208 = Dequeue Element(queue=w333) -> ()  [unwired: 2 in, 4 out]
        n209 = local read "threshold"() -> (w344:i32)
        n210 = local read "frames"() -> (w343:i32)
        n211 = local read "count?"() -> (w342:bool)
        n212 = local read "dark?"() -> (w345:bool)
        n213 = for {
          N: w343 -> [w359]
          tunnel: w345 -> [w371]
          tunnel: w336 -> [w369]
          tunnel: w341 -> [w370]
          tunnel: w344 -> [w363]
          tunnel: [w367] -> w337
          shift-right: [w366] -> w338
          shift-left: w340 -> [w368]
          tunnel: w339 -> [w362]
          tunnel: w342 -> [w361]
          tunnel: [w357] -> w335 mode=indexing
          shift-right: [w349] -> w325
          shift-left: w328 -> [w350]
          tunnel: w327 -> [w348]
          shift-right: [w346] -> w324
          shift-left: w326 -> [w347]
          i -> [w360]
          n214 = call "tm_getnextframe_a.vi"("error in (no error)"=w368, "Buffer"=w369, "Handle in"=w370) -> ("error out"=w366:errorcluster, "Data"=w365:u16[][], "Handle out"=w367:u32)  [unwired: 6 in]
          n215 = call "ringbuffer.vi"("index in"=w347, "array size"=w348, "array in"=w350) -> ("index out"=w346:i32, "array out"=w349:dbl[])  [unwired: 7 in]
          n216 = Divide(x=w360, y=w359) -> (x/y=w358:dbl)
          n217 = case shown="True" w371 {
            tunnel: [w372 w375] -> w364
            tunnel: w365 -> [w372 w374]
            tunnel: w362 -> [_ w373]
            frame False {
            }
            frame True {
              n218 = Subtract(x=w374, y=w373) -> (x-y=w375:dbl[][])
            }
          }
          n219 = local write "Slide"(w358) -> ()
          n220 = call <vilib>:"Std Deviation and Variance.vi"("X"=w349) -> ("mean"=w351:dbl, "standard deviation"=w354:dbl)  [unwired: 1 in, 1 out]
          n221 = call "filtr_b.vi"("count?"=w361, "threshold"=w363, "input array"=w364) -> ("output array"=w356:dbl[][])  [unwired: 8 in]
          n222 = Divide(x=w354, y=w351) -> (x/y=w353:dbl)
          n223 = local write "live"(w356) -> ()
          n224 = Multiply(x=w353, y=100.0) -> (x*y=w355:dbl)
          n225 = local write "noise-o-meter"(w355) -> ()
          n226 = Add Array Elements(numeric array=w356) -> (sum=w357:dbl)
          n227 = local write "Waveform Chart"(w357) -> ()
        }
        n228 = call <vilib>:"Std Deviation and Variance.vi"("X"=w335) -> ("mean"=w332:dbl, "standard deviation"=w331:dbl)  [unwired: 1 in, 1 out]
        n229 = Format Into String(format string="%.6e;%.6e", w332, w331) -> (resulting string=w330:string)  [unwired: 2 in, 1 out]
        n230 = Enqueue Element(queue=w334, element=w330) -> ()  [unwired: 2 in, 3 out]
      }
      frame "dark" {
        n231 = Dequeue Element(queue=w382) -> ()  [unwired: 2 in, 4 out]
        n232 = local read "captured"() -> (w378:dbl[][])
      }
      frame "dark_load" {
        n233 = Dequeue Element(queue=w392) -> ()  [unwired: 2 in, 4 out]
        n234 = String To Path(string=w388) -> (path=w387:path)
        n235 = Read from Binary File(5:dbl[][] [] ("all rows"), 11:w387) -> (2:w385:dbl[][])  [unwired: 4 in, 3 out]
        n236 = call-poly <vilib>:"Read From Spreadsheet File.vi"("file path (dialog if empty)"=w387) -> ()  [unwired: 6 in, 5 out]
      }
      frame "release" {
        n237 = call "tm_stopcapture.vi"("error in (no error)"=w400, "Handle in"=w401) -> ("error out"=w398:errorcluster, "Handle out"=w399:u32)  [unwired: 8 in]
        n238 = Dequeue Element(queue=w404) -> ()  [unwired: 2 in, 4 out]
        n239 = call "tm_closecamera.vi"("error in (no error)"=w398, "Handle in"=w399) -> ("error out"=w397:errorcluster)  [unwired: 9 in]
        n240 = call "tm_deinitialize.vi"("error in (no error)"=w397) -> ("error out"=w396:errorcluster)  [unwired: 10 in]
      }
      frame "init" {
        n241 = Dequeue Element(queue=w407) -> ()  [unwired: 2 in, 4 out]
        n242 = call "tm_initialize.vi"() -> ("error out"=w413:errorcluster)  [unwired: 8 in, 3 out]
        n243 = call "tm_opencamera.vi"("error in (no error)"=w413, "Camera Index"=u32 0) -> ("error out"=w412:errorcluster, "Handle out"=w410:u32)  [unwired: 7 in, 1 out]
      }
      frame "set" {
        w439 = 1 items=["Snap", "Sequence"] ("Capture mode")
        w440 = u32 4215968 items=["BINNING"=4215968, "BITS PER CHANNEL"=2, "ACTIVE VIEW INDEX"=3, "CCD MODE"=4, "SENSOR MODE"=5, "READOUT MODE"=6, "EXPOSURE TIME"=7, "CONTRAST GAIN"=8, "CONTRAST OFFSET"=9, "LIGHT MODE"=10, "SENSITIVITY"=11, "WHITE BALANCE"=12, "PHOTON IMAGING MODE"=13, "HIGH DYNAMIC RANGE MODE"=14, "TRIGGER SOURCE"=15, "TRIGGER ACTIVE"=16, "TRIGGER MODE"=17, "TRIGGER POLARITY"=18, "TRIGGER GLOBAL EXPOSURE"=19, "FIRST TRIGGER BEHAVIOR"=20, "TRIGGER TIMES"=21, "OUTPUT TRIGGER POLARITY"=22, "OUTPUT TRIGGER DELAY"=23, "OUTPUT TRIGGER PERIOD"=24, "TEMPERATURE"=25, "TEMPERATURE TARGET"=26, "SENSOR COOLER FAN"=27, "MECHANICAL SHUTTER"=28, "BACK FOCUS POSITION"=29, "FRAMEBUNDLE MODE"=30, "FRAMEBUNDLE NUMBER"=31, "LINEBUNDLE HEIGHT"=32, "TRIGGER CONNECTOR"=33, "IMAGE PIXEL TYPE"=34, "OUTPUT TRIGGER KIND"=35, "READOUT DIRECTION"=36, "CHANNEL SYNC"=37] ("Parameter")
        w417 = u32 7 items=["BINNING"=4215968, "BITS PER CHANNEL"=2, "ACTIVE VIEW INDEX"=3, "CCD MODE"=4, "SENSOR MODE"=5, "READOUT MODE"=6, "EXPOSURE TIME"=7, "CONTRAST GAIN"=8, "CONTRAST OFFSET"=9, "LIGHT MODE"=10, "SENSITIVITY"=11, "WHITE BALANCE"=12, "PHOTON IMAGING MODE"=13, "HIGH DYNAMIC RANGE MODE"=14, "TRIGGER SOURCE"=15, "TRIGGER ACTIVE"=16, "TRIGGER MODE"=17, "TRIGGER POLARITY"=18, "TRIGGER GLOBAL EXPOSURE"=19, "FIRST TRIGGER BEHAVIOR"=20, "TRIGGER TIMES"=21, "OUTPUT TRIGGER POLARITY"=22, "OUTPUT TRIGGER DELAY"=23, "OUTPUT TRIGGER PERIOD"=24, "TEMPERATURE"=25, "TEMPERATURE TARGET"=26, "SENSOR COOLER FAN"=27, "MECHANICAL SHUTTER"=28, "BACK FOCUS POSITION"=29, "FRAMEBUNDLE MODE"=30, "FRAMEBUNDLE NUMBER"=31, "LINEBUNDLE HEIGHT"=32, "TRIGGER CONNECTOR"=33, "IMAGE PIXEL TYPE"=34, "OUTPUT TRIGGER KIND"=35, "READOUT DIRECTION"=36, "CHANNEL SYNC"=37] ("Parameter")
        n244 = Dequeue Element(queue=w433) -> ()  [unwired: 2 in, 4 out]
        n245 = call "tm_stopcapture.vi"("error in (no error)"=w447, "Handle in"=w445) -> ("error out"=w446:errorcluster, "Handle out"=w444:u32)  [unwired: 8 in]
        n246 = call "tm_unpreparecapture.vi"("error in (no error)"=w446, "Handle in"=w444) -> ("error out"=w443:errorcluster, "Handle out"=w442:u32)  [unwired: 8 in]
        n247 = call "tm_setparameter.vi"("error in (no error)"=w443, "Value in"="t_exp", "Parameter"=w417, "Handle in"=w442) -> ("error out"=w419:errorcluster, "Handle out"=w418:u32)  [unwired: 6 in]
        n248 = call "tm_getparameter.vi"("error in (no error)"=w419, "Parameter"=w417, "Handle in"=w418) -> ("error out"=w415:errorcluster, "Value out"=w414:dbl, "Handle out"=w416:u32)  [unwired: 6 in]
        n249 = local write "t_exp"(w414) -> ()
        n250 = call "tm_setparameter.vi"("error in (no error)"=w415, "Value in"="Value in", "Parameter"=w440, "Handle in"=w416) -> ("error out"=w423:errorcluster, "Handle out"=w424:u32)  [unwired: 6 in]
        n251 = call "tm_preparecapture.vi"("error in (no error)"=w423, "Frames"=1, "Capture mode"=w439, "Handle in"=w424) -> ("error out"=w436:errorcluster, "Buffer Info"=w435:T4, "Handle out"=w437:u32)  [unwired: 4 in, 1 out]
        n252 = call "tm_startcapture_b.vi"("error in (no error)"=w436, "Handle in"=w437) -> ("error out"=w421:errorcluster, "Handle out"=w422:u32)  [unwired: 8 in]
        n253 = Unbundle(w435) -> ("height"=w431:u32, "width"=w432:u32)  [unwired: 1 out]
        n254 = property on="live" class="IntGraph (strict)"("XScale.Minimum"=0.0 ("X Scale.Range:Minimum"), "XScale.Maximum"=w431, "YScale.Minimum"=0.0 ("Y Scale.Range:Minimum"), "YScale.Maximum"=w432) -> ()  [unwired: 2 in, 2 out]
        n255 = Initialize Array(u16 0 ("element"), w431, w432) -> (w434:u16[][])
      }
      frame "close" {
        n256 = Release Queue(queue=w455) -> ()  [unwired: 2 in, 3 out]
      }
    }
  }
  n257 = while {
    shift-right: [w458] -> _
    shift-left: _ -> [w466]
    shift-right: [w464] -> _
    shift-left: 200 -> [w465]
    shift-right: [w462] -> _
    shift-left: _ -> [w461]
    tunnel: w20 -> [w459]
    tunnel: w17 -> [w456]
    stop <- w467 stop-if-true
    # "ESP301"
    n258 = Preview Queue Element(queue=w456, timeout in ms (-1)=w465) -> (queue out=w463:refnum<queue>, element=w471:string)  [unwired: 1 in, 2 out]
    n259 = Match Pattern(string=w471, regular expression=":") -> (before substring=w469:string, after substring=w468:string)  [unwired: 1 in, 2 out]
    n260 = case shown="\"abs\"" w469 {
      tunnel: w468 -> [_ w496 w536 _ _ _]
      tunnel: [_ _ _ _ _ TRUE] -> w467
      tunnel: [w480 w491 w532 w539 w547 w552] -> w458
      tunnel: w466 -> [w483 w500 w534 w541 _ w552]
      tunnel: w463 -> [_ w487 w528 w538 w548 w550]
      tunnel: [w481 w484 w533 refnum<visa-resource-name> refnum ("VISA resource name out") w546 w551] -> w462
      tunnel: w461 -> [w482 w499 w535 w542 _ w551]
      tunnel: "esp_axis" -> [w479 w485 w531 _ _ _]
      tunnel: w459 -> [_ w489 _ _ _ _]
      tunnel: [200 0 0 0 0 0] -> w457
      frame "idle", Default {
        n261 = call "Read Actual Position.vi"("error in (no error)"=w483, "Axis (1)"=w479, "VISA resource name"=w482) -> ("error out"=w480:errorcluster, "Position (units)"=w474:dbl, "VISA resource name out"=w481:refnum<visa-resource-name>)  [unwired: 2 in]
        n262 = local read "t0 @"() -> (w477:dbl)
        n263 = call "mm2time.vi"("fs?"=TRUE, "Offset (mm)"=w477, "distance (mm)"=w474) -> ("time in fs/ps seconds"=w475:dbl)
        n264 = local write "delay_pos"(w474) -> ()
        n265 = local write "esp_pos_fs"(w475) -> ()
      }
      frame "abs" {
        n266 = Dequeue Element(queue=w487) -> ()  [unwired: 2 in, 4 out]
        n267 = Match Pattern(string=w496, regular expression=":") -> (before substring=w495:string, after substring=w494:string)  [unwired: 1 in, 2 out]
        n268 = Equal?(x=w494, y="confirm") -> (x = y?=w490:bool)
        n269 = Fract/Exp String To Number(string=w495) -> (number=w498:dbl)  [unwired: 3 in, 1 out]
        n270 = call "Move Absolute.vi"("error in (no error)"=w500, "Position (0 units)"=w498, "Axis (1)"=w485, "VISA resource name"=w499) -> ("error out"=w492:errorcluster, "VISA resource name out"=w486:refnum<visa-resource-name>)  [unwired: 2 in]
        n271 = case shown="True" w490 {
          tunnel: w492 -> [w502 w507]
          tunnel: [w502 w510] -> w491
          tunnel: w489 -> [_ w509]
          tunnel: w486 -> [w501 w505]
          tunnel: w485 -> [_ w504]
          tunnel: [w501 w503] -> w484
          frame False {
          }
          frame True {
            n272 = while {
              tunnel: w505 -> [w515]
              tunnel: w504 -> [w511]
              shift-right: [w519] -> w506
              shift-left: w507 -> [w514]
              tunnel: [w518] -> w503
              stop <- w521 continue-if-true
              n273 = call "Read Actual Position.vi"("error in (no error)"=w514, "Axis (1)"=w511, "VISA resource name"=w515) -> ("error out"=w512:errorcluster, "Position (units)"=w516:dbl, "VISA resource name out"=w513:refnum<visa-resource-name>)  [unwired: 2 in]
              n274 = local write "delay_pos"(w516) -> ()
              n275 = Decrement(x=w511) -> (x-1=w517:i32)
              n276 = call "Get Controller Status.vi"("error in (no error)"=w512, "VISA resource name"=w513) -> ("error out"=w519:errorcluster, "Controller Status"=w527:T5, "VISA resource name out"=w518:refnum<visa-resource-name>)  [unwired: 2 in, 1 out]
              n277 = Unbundle(w527) -> ("Axis1 moving"=w526:bool, "Axis2 moving"=w525:bool, "Axis3 moving"=w524:bool, "Axis4 moving"=w523:bool)  [unwired: 12 out]
              n278 = Build Array(w526, w525, w524, w523) -> (w522:bool[])
              n279 = Index Array(array=w522, index=w517) -> (element=w520:bool)
              n280 = Or(x=w520, y=w519) -> (x .or. y?=w521:bool)
            }
            n281 = Send Notification(notification=TRUE, notifier=w509, error in (no error)=w506) -> (error out=w510:errorcluster)  [unwired: 1 out]
          }
        }
      }
      frame "rel" {
        n282 = Dequeue Element(queue=w528) -> ()  [unwired: 2 in, 4 out]
        n283 = Fract/Exp String To Number(string=w536) -> (number=w530:dbl)  [unwired: 3 in, 1 out]
        n284 = call "Move Relative.vi"("error in (no error)"=w534, "Position (0 units)"=w530, "Axis (1)"=w531, "VISA resource name"=w535) -> ("error out"=w532:errorcluster, "VISA resource name out"=w533:refnum<visa-resource-name>)  [unwired: 2 in]
      }
      frame "release" {
        n285 = Dequeue Element(queue=w538) -> ()  [unwired: 2 in, 4 out]
        n286 = call "Close.vi"("error in (no error)"=w541, "VISA resource name"=w542) -> ("error out"=w539:errorcluster)  [unwired: 9 in]
      }
      frame "init" {
        n287 = Dequeue Element(queue=w548) -> ()  [unwired: 2 in, 4 out]
        n288 = call "Initialize.vi"("VISA resource name"="esp_visa", "Serial Link (RS232)"="Serial Link (RS232)") -> ("VISA resource name out"=w546:refnum<visa-resource-name>, "error out"=w547:errorcluster)  [unwired: 7 in]
      }
      frame "close" {
        n289 = Release Queue(queue=w550) -> ()  [unwired: 2 in, 3 out]
      }
    }
    "esp301" <- w458
    n290 = case shown="No Error" w458 {
      tunnel: [w472 -1] -> w464
      tunnel: w457 -> [w472 _]
      frame No Error {
      }
      frame Error {
      }
    }
  }
  n291 = while {
    tunnel: w25 -> [w562]
    shift-right: [w560] -> _
    shift-left: _ -> [w559]
    shift-right: [w557] -> _
    shift-left: -1 -> [w558]
    shift-right: [w556] -> _
    shift-left: _ -> [w555]
    tunnel: w23 -> [w554]
    stop <- w561 stop-if-true
    # "ISEG"
    n292 = Preview Queue Element(queue=w562, timeout in ms (-1)=w558) -> (element=w566:string)  [unwired: 1 in, 3 out]
    n293 = Match Pattern(string=w566, regular expression=":") -> (before substring=w564:string, after substring=w563:string)  [unwired: 1 in, 2 out]
    n294 = case shown="\"set\"" w564 {
      tunnel: w563 -> [_ w580 _ _ _]
      tunnel: w562 -> [_ w592 w634 w638 w642]
      tunnel: [_ _ _ _ TRUE] -> w561
      tunnel: [w569 w586 w632 w637 w639] -> w560
      tunnel: w559 -> [w571 w590 _ _ w639]
      tunnel: [0 _ _ _ _] -> w557
      tunnel: [w570 w587 T6 {"VISA Resource Name"="", "FP Notation"=FALSE, "Maximum Voltage"=0, "Maximum Current"=0} ("VISA Session Out") w635 w640] -> w556
      tunnel: w555 -> [w572 w591 w633 _ w640]
      tunnel: w554 -> [_ w575 _ _ _]
      frame "idle", Default {
        n295 = local read "Channel (A)"() -> (w573:enum16{"A", "B"})
        n296 = call "iseg NHQ xxx GetActualVoltage.vi"("error in (no error)"=w571, "Channel (A)"=w573, "VISA Session"=w572) -> ("error out"=w569:errorcluster, "Voltage"=w568:dbl, "VISA Session Out"=w570:T6)  [unwired: 5 in, 1 out]
        n297 = node(w568) -> (w567:dbl[unit])
        n298 = local write "Actual Voltage"(w567) -> ()
      }
      frame "set" {
        n299 = local read "Channel (A)"() -> (w583:enum16{"A", "B"})
        n300 = Dequeue Element(queue=w592) -> ()  [unwired: 2 in, 4 out]
        n301 = Match Pattern(string=w580, regular expression=":") -> (before substring=w579:string, after substring=w578:string)  [unwired: 1 in, 2 out]
        n302 = Fract/Exp String To Number(string=w579) -> (number=w582:dbl)  [unwired: 3 in, 1 out]
        n303 = call "iseg NHQ xxx SetNominalVoltage.vi"("error in (no error)"=w590, "Voltage (0 V)"=w582, "Channel (A)"=w583, "VISA Session"=w591) -> ("error out"=w593:errorcluster, "VISA Session Out"=w594:T6)  [unwired: 6 in]
        n304 = Equal?(x=w578, y="wait") -> (x = y?=w576:bool)
        n305 = call "iseg NHQ xxx StartVoltageChange.vi"("error in (no error)"=w593, "Channel (A)"=w583, "VISA Session"=w594) -> ("error out"=w588:errorcluster, "VISA Session Out"=w589:T6)  [unwired: 6 in, 1 out]
        n306 = case shown="True" w576 {
          tunnel: [w596 w606] -> w587
          tunnel: [w595 w598] -> w586
          tunnel: w589 -> [w596 w605]
          tunnel: w588 -> [w595 w604]
          tunnel: w582 -> [_ w603]
          tunnel: "volt_threshold" -> [_ w602]
          tunnel: "volt_timeout" -> [_ w601]
          tunnel: w583 -> [_ w600]
          tunnel: w575 -> [_ w599]
          frame False {
          }
          frame True {
            n307 = Tick Count (ms)() -> (millisecond timer value=w607:u32)
            n308 = while {
              shift-right: [w628] -> w606
              shift-left: w605 -> [w630]
              shift-right: [w615] -> w598
              shift-left: w604 -> [w629]
              tunnel: w600 -> [w627]
              tunnel: w602 -> [w624]
              tunnel: w607 -> [w622]
              tunnel: w601 -> [w620]
              tunnel: w603 -> [w619]
              tunnel: [w610] -> w597
              stop <- w616 stop-if-true
              n309 = Tick Count (ms)() -> (millisecond timer value=w623:u32)
              n310 = call "iseg NHQ xxx GetActualVoltage.vi"("error in (no error)"=w629, "Channel (A)"=w627, "VISA Session"=w630) -> ("error out"=w615:errorcluster, "Voltage"=w608:dbl, "VISA Session Out"=w628:T6)  [unwired: 5 in, 1 out]
              n311 = Absolute Value(x=w608) -> (abs(x)=w618:dbl)
              n312 = node(w608) -> (w609:dbl[unit])
              n313 = Subtract(x=w623, y=w622) -> (x-y=w621:u32)
              n314 = Subtract(x=w618, y=w619) -> (x-y=w626:dbl)
              n315 = local write "Actual Voltage"(w609) -> ()
              n316 = Absolute Value(x=w626) -> (abs(x)=w625:dbl)
              n317 = Greater?(x=w621, y=w620) -> (0:w614:bool)
              n318 = Less?(x=w625, y=w624) -> (x < y?=w617:bool)
              n319 = Or(x=w615, y=w614) -> (x .or. y?=w613:bool)
              n320 = Compound Arithmetic op=OR(w615, w617, w614) -> (w616:bool)
              n321 = Select(t="fail" ("element"), s=w613, f="done" ("element")) -> (s? t:f=w610:string)
            }
            n322 = Enqueue Element(queue=w599, element=w597) -> ()  [unwired: 2 in, 3 out]
          }
        }
      }
      frame "release" {
        n323 = Dequeue Element(queue=w634) -> ()  [unwired: 2 in, 4 out]
        n324 = call "iseg NHQ xxx Close.vi"("VISA session"=w633) -> ("error out"=w632:errorcluster)  [unwired: 14 in]
      }
      frame "init" {
        n325 = Dequeue Element(queue=w638) -> ()  [unwired: 2 in, 4 out]
        n326 = call "iseg NHQ xxx Initialize.vi"("VISA resource name"="VISA ISEG") -> ("VISA Session Out"=w635:T6, "error out"=w637:errorcluster)  [unwired: 13 in]
      }
      frame "close" {
        n327 = Release Queue(queue=w642) -> ()  [unwired: 2 in, 3 out]
      }
    }
    "error out" <- w560
  }
  n328 = while {
    tunnel: w23 -> [w651]
    tunnel: w31 -> [w650]
    tunnel: w30 -> [w648]
    tunnel: w25 -> [w647]
    tunnel: w6 -> [w646]
    tunnel: w20 -> [w645]
    tunnel: w17 -> [w644]
    tunnel: w1 -> [w643]
    stop <- w649 stop-if-true
    # "coherent"
    n329 = Preview Queue Element(queue=w651) -> (element=w655:string)  [unwired: 2 in, 3 out]
    n330 = Match Pattern(string=w655, regular expression=":") -> (before substring=w653:string, after substring=w652:string)  [unwired: 1 in, 2 out]
    n331 = case shown="\"delay\"" w653 {
      tunnel: w652 -> [_ _ _ _ _]
      tunnel: w651 -> [w657 w663 w688 w773 _]
      tunnel: w650 -> [w658 w659 w680 w771 _]
      tunnel: [TRUE _ _ _ _] -> w649
      tunnel: w648 -> [_ w662 w681 w770 _]
      tunnel: w647 -> [_ _ w682 _ _]
      tunnel: w646 -> [_ _ w683 _ _]
      tunnel: w645 -> [_ _ _ w787 _]
      tunnel: w644 -> [_ _ _ w768 _]
      tunnel: w643 -> [_ _ _ _ _]
      frame "close" {
        n332 = Release Queue(queue=w657) -> ()  [unwired: 2 in, 3 out]
        n333 = Release Queue(queue=w658) -> ()  [unwired: 2 in, 3 out]
      }
      frame "single" {
        n334 = Dequeue Element(queue=w663) -> (error out=w660:errorcluster)  [unwired: 2 in, 3 out]
        n335 = Flush Queue(queue=w659, error in (no error)=w660) -> (error out=w661:errorcluster)  [unwired: 2 out]
        n336 = while {
          tunnel: w662 -> [w667]
          tunnel: w661 -> [w666]
          tunnel: w659 -> [w665]
          stop <- w664 continue-if-true
          n337 = flat-sequence {
            tunnel: w667 -> [w672]
            tunnel: w666 -> [w669]
            tunnel: w665 -> [w668]
            tunnel: ["continous acq."] -> w664
            frame #0 {
              n338 = Enqueue Element(queue=w672, element="snap", error in (no error)=w669) -> (error out=w670:errorcluster)  [unwired: 1 in, 2 out]
              n339 = Dequeue Element(queue=w668, error in (no error)=w670) -> ()  [unwired: 1 in, 4 out]
            }
            frame #1 {
            }
          }
        }
      }
      frame "volt" {
        n340 = Flush Queue(queue=w688) -> (queue out=w684:refnum<queue>)  [unwired: 1 in, 2 out]
        n341 = local read "Path"() -> (w687:path)
        n342 = Build Path(base path=w687, name or relative path="head") -> (appended path=w675:path)
        n343 = Build Path(base path=w675, name or relative path="raw") -> (appended path=w677:path)
        n344 = Build Path(base path=w675, name or relative path="LUT.txt") -> (appended path=w678:path)
        n345 = Create Folder(path (use dialog)=w677) -> (created path=w676:path)  [unwired: 2 in, 2 out]
        n346 = while {
          tunnel: w684 -> [w689]
          tunnel: w683 -> [w712]
          tunnel: w682 -> [w706]
          tunnel: w681 -> [w705]
          tunnel: w680 -> [w704]
          tunnel: w678 -> [w699]
          tunnel: w676 -> [w698]
          shift-right: [w691] -> _
          shift-left: _ -> [w696]
          tunnel: [w689] -> w674
          i -> [w703]
          stop <- w690 stop-if-true
          n347 = call-poly <vilib>:"Ramp Pattern.vi"("start"="volt_start", "end"="volt_end", "samples"="volt_samples") -> ("Ramp Pattern"=w702:dbl[])  [unwired: 7 in, 1 out]
          n348 = Array Size(array=w702) -> (size(s)=w701:i32)
          n349 = Number To Fractional String(number=w702) -> (F-format string=w708:string[])  [unwired: 3 in]
          n350 = Multiply(x=w701, y=w703) -> (x*y=w700:i32)
          n351 = for {
            N -> [w715]
            tunnel: w712 -> [w742]
            tunnel: w689 -> [w749]
            tunnel: w708 -> [w732] mode=indexing
            tunnel: "set:" ("element") -> [w746]
            tunnel: w706 -> [w745]
            tunnel: w689 -> [w743]
            tunnel: w705 -> [w740]
            tunnel: w704 -> [w737]
            shift-right: [w717] -> w697
            shift-left: w696 -> [w735]
            tunnel: w700 -> [w734]
            tunnel: w699 -> [w731]
            tunnel: w698 -> [w730]
            tunnel: ":wait" ("element") -> [w716]
            i -> [w714]
            n352 = Concatenate Strings(w746, w732, w716) -> (w747:string)
            n353 = Add(x=w734, y=w714) -> (x+y=w733:i32)
            n354 = Divide(x=w714, y=w715) -> (x/y=→"Slide 2":dbl)
            n355 = Number To Decimal String(number=w733) -> (decimal integer string=w729:string)  [unwired: 1 in]
            n356 = Enqueue Element(queue=w745, element=w747, error in (no error)=w735) -> (error out=w744:errorcluster)  [unwired: 1 in, 2 out]
            n357 = Dequeue Element(queue=w743, error in (no error)=w744) -> (element=w726:string, error out=w724:errorcluster)  [unwired: 1 in, 2 out]
            n358 = Equal?(x="stop" ("y"), y=w726) -> (x = y?=w723:bool)
            n359 = call "inject_error.vi"("error in"=w724, "s"=w723) -> ("error out"=w725:errorcluster)  [unwired: 9 in]
            n360 = Enqueue Element(queue=w742, element="start", error in (no error)=w725) -> (error out=w739:errorcluster)  [unwired: 1 in, 2 out]
            n361 = Enqueue Element(queue=w740, element="snap", error in (no error)=w739) -> (error out=w738:errorcluster)  [unwired: 1 in, 2 out]
            n362 = Dequeue Element(queue=w737, error in (no error)=w738) -> (element=w728:dbl[][], error out=w736:errorcluster)  [unwired: 1 in, 2 out]
            n363 = Enqueue Element(queue=w742, element="ok", error in (no error)=w736) -> (error out=w748:errorcluster)  [unwired: 1 in, 2 out]
            n364 = Dequeue Element(queue=w749, error in (no error)=w748) -> (element=w720:string, error out=w719:errorcluster)  [unwired: 1 in, 2 out]
            n365 = Equal?(x="stop" ("y"), y=w720) -> (x = y?=w722:bool)
            n366 = call "inject_error.vi"("error in"=w719, "s"=w722) -> ("error out"=w718:errorcluster)  [unwired: 9 in]
            n367 = case shown="No Error" w718 {
              selector: w718 -> [w755 w765]
              tunnel: w732 -> [w754 _]
              tunnel: w731 -> [w761 _]
              tunnel: w730 -> [w760 _]
              tunnel: w729 -> [w759 _]
              tunnel: w728 -> [w757 _]
              tunnel: w720 -> [w756 _]
              tunnel: [w755 w765] -> w717
              frame No Error {
                n368 = Build Path(base path=w760, name or relative path=w759) -> (appended path=w758:path)
                n369 = Match Pattern(string=w756, regular expression=";") -> (before substring=w762:string, after substring=w753:string)  [unwired: 1 in, 2 out]
                n370 = Write to Binary File(file (use dialog)=w758, data=w757) -> ()  [unwired: 4 in, 3 out]
                n371 = Build Array(w759, w762, w753, w754) -> (w752:string[])
                n372 = call-poly <vilib>:"Write Delimited Spreadsheet.vi"("file path (dialog if empty)"=w761, "1D data"=w752, "append to file? (new file:F)"=TRUE) -> ()  [unwired: 11 in, 2 out]
              }
              frame Error {
              }
            }
          }
          n373 = Dequeue Element(queue=w689, error in (no error)=w697) -> (element=w694:string, error out=w691:errorcluster)  [unwired: 1 in, 2 out]
          n374 = Equal?(x="stop" ("y"), y=w694) -> (x = y?=w692:bool)
          n375 = Or(x=w692, y=w691) -> (x .or. y?=w690:bool)
        }
        n376 = Flush Queue(queue=w674) -> ()  [unwired: 1 in, 3 out]
      }
      frame "delay" {
        n377 = local read "Path"() -> (w786:path)
        n378 = Dequeue Element(queue=w773) -> ()  [unwired: 2 in, 4 out]
        n379 = Build Path(base path=w786, name or relative path="delayscan_header") -> (appended path=w775:path)
        n380 = call <vilib>:"Check if File or Folder Exists.vi"("path"=w775) -> ("file or folder exists?"=w777:bool, "dup path"=w776:path)  [unwired: 8 in, 1 out]
        n381 = case shown="False" w777 {
          tunnel: [w919 w920] -> w774
          tunnel: w776 -> [w918 w920]
          frame False {
            n382 = Create Folder(path (use dialog)=w918) -> (created path=w919:path)  [unwired: 2 in, 2 out]
          }
          frame True {
          }
        }
        n383 = call "create scan vectr.vi"("Table Control"="waypoints") -> ("Array"=w778:dbl[])
        n384 = Flush Queue(queue=w771) -> (queue out=w772:refnum<queue>)  [unwired: 1 in, 2 out]
        n385 = Array Size(array=w778) -> (size(s)=w781:i32)
        n386 = Build Path(base path=w774, name or relative path="times.txt") -> (appended path=w783:path)
        n387 = Flush Queue(queue=w768) -> (queue out=w767:refnum<queue>)  [unwired: 1 in, 2 out]
        n388 = Flush Queue(queue=w770) -> (queue out=w769:refnum<queue>)  [unwired: 1 in, 2 out]
        n389 = Get Date/Time In Seconds() -> (seconds since 1Jan1904=w766:timestamp)
        n390 = Initialize Array(0.0 ("element"), w781) -> (w779:dbl[])
        n391 = call-poly <vilib>:"Write Delimited Spreadsheet.vi"("file path (dialog if empty)"=w783, "1D data"=w778, "transpose? (no:F)"=TRUE) -> ()  [unwired: 11 in, 2 out]
        n392 = while {
          tunnel: w778 -> [w800]
          tunnel: w767 -> [w804]
          tunnel: w787 -> [w803]
          tunnel: w772 -> [w802]
          tunnel: w769 -> [w801]
          tunnel: w774 -> [w799]
          shift-right: [w797] -> _
          shift-left: w779 -> [w798]
          tunnel: w774 -> [w796]
          tunnel: w766 -> [w790]
          i -> [w794]
          stop <- w791 stop-if-true
          n393 = for {
            N -> [w815]
            tunnel: w800 -> [w821] mode=indexing
            tunnel: w804 -> [w885]
            tunnel: w803 -> [w883]
            tunnel: w802 -> [w881]
            tunnel: w801 -> [w879]
            tunnel: w800 -> [w849]
            tunnel: w799 -> [w877]
            tunnel: w794 -> [w819]
            shift-right: [w847] -> w797
            shift-left: w798 -> [w850]
            tunnel: w796 -> [w845]
            tunnel: [w820] -> w793
            tunnel: w790 -> [w813]
            tunnel: "iterations" -> [w816]
            i -> [w811]
            stop <- w820 stop-if-true
            n394 = Multiply(x=w815, y=w819) -> (x*y=w818:i32)
            n395 = local read "t0 @"() -> (w890:dbl)
            n396 = Get Date/Time In Seconds() -> (seconds since 1Jan1904=w817:timestamp)
            n397 = Get Date/Time In Seconds() -> (seconds since 1Jan1904=w826:timestamp)
            n398 = Add(x=w818, y=w811) -> (x+y=w805:i32)
            n399 = Divide(x=w819, y=10000) -> (x/y=w875:dbl)
            n400 = Subtract(x=w813, y=w817) -> (x-y=w814:dbl)
            n401 = Format Date/Time String(time format string (%c)="DelayScan_%Y%m%d_%H%M%S_", seconds (now)=w826) -> (date/time string=w822:string)  [unwired: 1 in]
            n402 = Divide(x=w814, y=w805) -> (x/y=w809:dbl)
            n403 = Multiply(x=w816, y=w815) -> (x*y=w812:i32)
            n404 = Divide(x=w811, y=10000) -> (x/y=w832:dbl)
            n405 = Number To Fractional String(number=w875) -> (F-format string=w874:string)  [unwired: 3 in]
            n406 = call "time2mm.vi"("fs[1]/ps[0]"=TRUE, "Offset (mm)"=w890, "time"=w821) -> ("position (mm)"=w829:dbl)
            n407 = Number To Fractional String(number=w832) -> (F-format string=w870:string)  [unwired: 3 in]
            n408 = Subtract(x=w812, y=w805) -> (x-y=w810:i32)
            n409 = local write "delayscan_time/step"(w809) -> ()
            n410 = Multiply(x=w809, y=w810) -> (x*y=w808:dbl)
            n411 = Number To Fractional String(number=w829) -> (F-format string=w888:string)  [unwired: 3 in]
            n412 = String Subset(string=w874, offset (0)=2, length (rest)=4 ("length (rest)")) -> (substring=w872:string)
            n413 = local write "duration"(w808) -> ()
            n414 = String Subset(string=w870, offset (0)=2, length (rest)=4 ("length (rest)")) -> (substring=w824:string)
            n415 = Concatenate Strings("abs:" ("string"), w888, ":confirm" ("string")) -> (w886:string)
            n416 = Build Path(base path=w877, name or relative path=w872) -> (appended path=w835:path)
            n417 = call <vilib>:"Check if File or Folder Exists.vi"("path"=w835) -> ("file or folder exists?"=w836:bool, "dup path"=w837:path)  [unwired: 8 in, 1 out]
            n418 = Concatenate Strings(w822, w824) -> (w825:string)
            n419 = case shown="False" w836 {
              tunnel: [w916 w917] -> w834
              tunnel: w837 -> [w915 w917]
              frame False {
                n420 = Create Folder(path (use dialog)=w915) -> (created path=w916:path)  [unwired: 2 in, 2 out]
              }
              frame True {
              }
            }
            n421 = Enqueue Element(queue=w885, element=w886) -> (error out=w884:errorcluster)  [unwired: 2 in, 2 out]
            n422 = Concatenate Strings(w825, ".bin" ("string")) -> (w841:string)
            n423 = Concatenate Strings(w825, ".png" ("string")) -> (w839:string)
            n424 = Wait on Notification(notifier=w883, error in (no error)=w884) -> (error out=w882:errorcluster)  [unwired: 2 in, 3 out]
            n425 = Build Path(base path=w834, name or relative path=w841) -> (appended path=w846:path)
            n426 = Build Path(base path=w845, name or relative path="positions.txt") -> (appended path=w843:path)
            n427 = property on="live" class="IntGraph (strict)"() -> ("CrsrLis"=w869:T7)  [unwired: 2 in, 2 out]
            n428 = Build Path(base path=w834, name or relative path=w839) -> (appended path=w838:path)
            n429 = Enqueue Element(queue=w879, element="snap", error in (no error)=w882) -> (error out=w880:errorcluster)  [unwired: 1 in, 2 out]
            n430 = Index Array(array=w869) -> (element #1=w868:T8, element #2=w867:T8)  [unwired: 2 in]
            n431 = Unbundle By Name(w868) -> ("Position.X"=w866:dbl, "Position.Y"=w864:dbl)
            n432 = Unbundle By Name(w867) -> ("Position.X"=w865:dbl, "Position.Y"=w863:dbl)
            n433 = Dequeue Element(queue=w881, error in (no error)=w880) -> (element=w807:dbl[][])  [unwired: 1 in, 3 out]
            n434 = Build Array(w866, w865) -> (w862:dbl[])
            n435 = Build Array(w864, w863) -> (w861:dbl[])
            n436 = Array Max & Min(array=w862) -> (max value=w860:dbl, min value=w858:dbl)  [unwired: 2 out]
            n437 = Array Max & Min(array=w861) -> (max value=w859:dbl, min value=w856:dbl)  [unwired: 2 out]
            n438 = while {
              tunnel: ["delayscan_stop"] -> w820
              tunnel: w807 -> [w892]
              tunnel: [w892] -> w806
              stop <- "delayscan_pause" continue-if-true
              n439 = Wait (ms)(milliseconds to wait=u32 100) -> ()  [unwired: 1 out]
            }
            n440 = Write to Binary File(file (use dialog)=w846, data=w806) -> ()  [unwired: 4 in, 3 out]
            n441 = Subtract(x=w858, y=w860) -> (x-y=w857:dbl)
            n442 = Subtract(x=w856, y=w859) -> (x-y=w855:dbl)
            n443 = Array Subset(array=w806, index (row)=w858, length (row)=w857, index (col)=w856, length (col)=w855) -> (w854:dbl[][])
            n444 = Array Size(array=w806) -> (size(s)=w852:i32[])
            n445 = Add Array Elements(numeric array=w854) -> (sum=w853:dbl)
            n446 = Multiply Array Elements(1:w852) -> (0:w851:i32)
            n447 = Divide(x=w853, y=w851) -> ()  [unwired: 1 out]
            n448 = disable-structure shown="Disabled" {
              disable-tunnel: w838 -> [w897 _]
              disable-tunnel: w806 -> [w896 _]
              frame Disabled {
                w911 = T2 7 items=["Grayscale (U8)", "Grayscale (I16)", "Grayscale (SGL)", "Complex (CSG)", "RGB (U32)", "HSL (U32)", "RGB (U64)", "Grayscale (U16)"] ("Image Type")
                n449 = for {
                  tunnel: w896 -> [w914] mode=indexing
                  tunnel: [w913] -> w906 mode=indexing
                  n450 = Reverse 1D Array(array=w914) -> (reversed array=w913:dbl[])
                }
                n451 = Transpose 2D Array(2D array=w906) -> (transposed array=w900:dbl[][])
                n452 = Array Max & Min(array=w900) -> (min value=w899:dbl)  [unwired: 3 out]
                n453 = Subtract(x=w900, y=w899) -> (x-y=w898:dbl[][])
                n454 = call "IMAQ Create"("Image Name"="untitled", "Image Type"=w911) -> ("New Image"=w912:T3)  [unwired: 3 in, 1 out]
                n455 = Array Max & Min(array=w898) -> (max value=w905:dbl)  [unwired: 3 out]
                n456 = Divide(x=w898, y=w905) -> (x/y=w904:dbl[][])
                n457 = Multiply(x=w904, y=255) -> (x*y=w902:dbl[][])
                n458 = To Unsigned Word Integer(number=w902) -> (unsigned 16bit integer=w901:u16[][])
                n459 = call "IMAQ ArrayToImage"("Image Pixels (U16)"=w901, "Image"=w912) -> ("Image Out"=w910:T3)  [unwired: 8 in, 1 out]
                n460 = call-poly "IMAQ Write File 2"("Image Quality"=u32 1000, "File Path"=w897, "Image"=w910) -> ("Image Out (duplicate)"=w908:T3)  [unwired: 7 in, 1 out]
                n461 = call "IMAQ Dispose"("Image"=w908) -> ()  [unwired: 5 in, 1 out]
              }
              frame Enabled {
              }
            }
            n462 = Replace Array Subset(array=w850, new element=w829, index=w811) -> (w847:dbl[])
            n463 = Bundle("Array"=w849, w847) -> (→"XY Graph":cluster{"Array":dbl[], dbl[]})  [unwired: 1 in]
            n464 = call-poly <vilib>:"Write Delimited Spreadsheet.vi"("file path (dialog if empty)"=w843, "format (%.3f)"="%.6f", "1D data"=w847, "transpose? (no:F)"=TRUE) -> ()  [unwired: 10 in, 2 out]
          }
          n465 = Increment(x=w794) -> (x+1=w795:i32)
          n466 = Greater Or Equal?(x=w795, y="iterations") -> (x >= y?=w792:bool)
          n467 = Or(x=w793, y=w792) -> (x .or. y?=w791:bool)
        }
      }
      frame "idle", Default {
      }
    }
  }
